vi "main.vi"() -> ()   [LabVIEW 2020]
uses:
  <vilib>/userDefined/High Color/IMAQdx.ctl
  Supporting Files/Sensor Station States.ctl
  Keyence CL-3000/Public/clusters/CL3IF_MEASUREMENT_DATA.ctl
  Keyence CL-3000/Public/clusters/CL3IF_OUTMEASUREMENT_DATA.ctl
  Keyence CL-3000/Public/enums/CL3IF_VALUE_INFO.ctl
  Keyence CL-3000/Public/enums/CL3IF_JUDGE_RESULT.ctl
  Keyence CL-3000/Public/clusters/CL3IF_ETHERNET_SETTING.ctl
  4961857f-4cb1-4452-8877-0132d1278599.vi
  4c07c87f-dbbe-4e69-95de-30caa6fe1779.vi
  8fbe439c-06e5-460e-a560-e938ce784f44.vi
  460a15f0-0b3a-4794-87ef-3f3f720a4f09.vi
  13309ec4-5ddb-4caa-9ccb-149c6c5ba2b7.vi
  762e2a81-f67b-4e5d-a3cd-0f967e3c6027.vi
  <vilib>/Utility/inputDevices.llb/keyboardAcquire.vi
  <vilib>/Utility/inputDevices.llb/closeKeyboard.vi
  Keyence CL-3000/Keyence CL-3000.lvlib
  <vilib>/vision/driver/NI_Vision_Acquisition_Software.lvlib
panel:
  in  "STOP":bool
  in  "Display Tab":enum32{"SENSOR FEEDBACK"}(tab)
  out "Chromatic Confocal":dbl(graph)
  out "Laser Displacement (cRIO)":dbl(graph)
  out "Captured Image":T1(plugin-control)
  out "Camera Feed":T1(plugin-control)
  in  "Motion Tab":enum32{"POSITION", "MEASUREMENT"}(tab)
  in  "Run Program":bool
  in  "Select Program":string(combo)="NONE"
  out "1st Key":T2(ring)
  in  "Bottom Button":bool
  in  "Top Button":bool
  in  "Next Button":bool
  in  "Previous Button":bool
  in  "Up Button":bool
  in  "Down Button":bool
  in  "Jog Axes":bool
  in  "Menu Ring":string(combo)
  in  "Move":bool
  in  "Axis 2 Distance":dbl format="%.2g"
  in  "Axis 1 Distance":dbl format="%.2g"
  in  "Axis 0 Distance":dbl format="%.2g"
  in  "Axis 0 Speed":dbl format="%.2g"
  in  "Axis 1 Speed":dbl format="%.2g"
  in  "Axis 2 Speed":dbl format="%.2g"
  in  "Axis 1 Acc":dbl format="%.2g"
  in  "Axis 0 Acc":dbl format="%.2g"
  in  "Axis 2 Acc":dbl format="%.2g"
  in  "Set Parameters 2":bool
  in  "Axis 2 Jogspeed":dbl format="%.2g"
  in  "Axis 1 Jogspeed":dbl format="%.2g"
  in  "Axis 0 Jogspeed":dbl format="%.2g"
  out "Laser Data Logged":i32
  in  "Capture Image":bool
  in  "Sensor":i32(ring) items=["Chromatic", "Laser"]
  in  "Chromatic Data \nLogging":bool
  out "Chromatic Data Logged":u32
  out "Index End":u32
  out "Index Start":u32
  out "Suffix":string
  in  "Measurement\nAxis":i32(ring) items=["X Axis", "Y Axis"]
  in  "Travel Speed\n(mm/s)":dbl format="%.2g"
  in  "Set Parameters":bool
  in  "Track Offset\n(mm)":dbl format="%.2g"
  in  "Ramp Distance\n(mm)":dbl min=0.0 format="%.2g"
  in  "Num Tracks":i32
  in  "Evaluation Length\n(mm)":dbl max=40.0 format="%.2g"
  in  "Test Name":string
  out "Laser Data\nLogging":bool
  out "Travel Dist":dbl
  in  "Travel Acc\n(mm/s2)":dbl format="%.2g"
  in  "Start Measurement":bool
  in  "Setup Tab":enum32{"SETUP", "MONITORING", "ERRORS"}(tab)
  in  "Home Axes":bool
  in  "Enable Camera":bool
  in  "Enable Laser":bool
  in  "Camera Input":T3
  in  "Enable Chromatic":bool
  in  "IP Address":u8[](array[numeric])=[192, 168, 1, 1]
  in  "Port":u32
  in  "Timeout":u32=5000
  in  "Comm Interface":enum8{"USB", "ETHERNET"}(ring)
  in  "Device ID":i32 min=0 max=2
  out "IsOpen":bool
  in  "Connection?":refnum<k7>(container)
  in  "Connect  to Controller":bool=TRUE
  in  "Set Parameters":bool
  in  "Controller Connection Type":string(combo)="2"
  out "Controller Type":string
  out "Product Name":string
  out "Version":string
  out "Serial Port":fxp<+,3,3>
  in  "Axis Enable":bool
  in  "Save Directory":path
  out "Z Error":bool
  out "Y Error":bool
  out "X Error":bool
  out "Axis 2 Velocity":dbl format="%.3g"
  out "Axis 2 End Pos":dbl format="%.3g"
  out "Axis 2 Position":dbl format="%.3g"
  out "Axis 0 Position":dbl format="%.3f"
  out "Axis 0 End Pos":dbl format="%.3g"
  out "Axis 0 Velocity":dbl format="%.3g"
  out "Axis 1 Position":dbl format="%.3g"
  out "Axis 1 Velocity":dbl format="%.3g"
  out "Axis 1 End Pos":dbl format="%.3g"
  out "A0 Remaining":dbl format="%.3g"
  out "A1 Remaining":dbl format="%.3g"
  out "A2 Remaining":dbl format="%.3g"
  out "Loop Time (us)":u32
  out "Measurement Data":T4(array[cluster])=[{"Out No"=1, "Value"=0, "valueInfo"=enum."VALID", "judgeResult"=0}, {"Out No"=2, "Value"=0, "valueInfo"=enum."VALID", "judgeResult"=0}, {"Out No"=3, "Value"=0, "valueInfo"=enum."VALID", "judgeResult"=0}, {"Out No"=4, "Value"=0, "valueInfo"=enum."VALID", "judgeResult"=0}, {"Out No"=5, "Value"=0, "valueInfo"=enum."VALID", "judgeResult"=0}, {"Out No"=6, "Value"=0, "valueInfo"=enum."VALID", "judgeResult"=0}, {"Out No"=7, "Value"=0, "valueInfo"=enum."VALID", "judgeResult"=0}, {"Out No"=8, "Value"=0, "valueInfo"=enum."VALID", "judgeResult"=0}] {"judgeResult" items=["HI"=1, "GO"=2, "LO"=4, "**"=5, "--"=0]}
  out "Total Time Elapsed (s)":i32
  out "XY Graph":cluster{"X":dbl, "Y":dbl}[](graph)
  out "Controller  Error":errorcluster
  out "Z Axis Error":errorcluster
  out "Y Axis Error":errorcluster
  out "X Axis Error":errorcluster
  out "Chromatic Sensor Error":errorcluster
  # "SET PARAMETERS"
  # "DIRECT MOTION"
  # "SPEED \n(mm/s)"
  # "ACC / DEC\n(mm/s2)"
  # "JOGSPEED \n(mm/s)"
  # "X AXIS"
  # "X AXIS"
  # "(mm)"
  # "Y AXIS"
  # "Y AXIS"
  # "(mm)"
  # "Z AXIS"
  # "Z AXIS"
  # "(mm)"
  # "AXIS JOGGING"
  # "XY AXES"
  # "Z AXIS"
  # "KEYBOARD"
  # "CONTROLLER PROGRAMS"
  # "Suffix will be auto-genereated for each measurement e.g. Test Name_01, Test Name_02, etc."
  # "MEASUREMENT PARAMETERS"
  # "CHROMATIC CONFOCAL"
  # "LASER DISPLACEMENT"
  # "CAMERA"
  # "CONTROLLER SETTINGS"
  # "CHROMATIC CONFOCAL SETTINGS"
  # "LASER DISPLACEMENT SETTINGS"
  # "CAMERA SETTINGS"
  # "AXIS FEEDBACK"
  # "Current Position \n(mm)"
  # "End Position \n(mm)"
  # "Travel Remaining \n(mm)"
  # "Velocity \n(mm/s2)"
  # "X AXIS"
  # "Y AXIS"
  # "Z AXIS"
  # "CONTROLLER"
  # "CHROMATIC CONFOCAL"
  # "CONTROLLER"
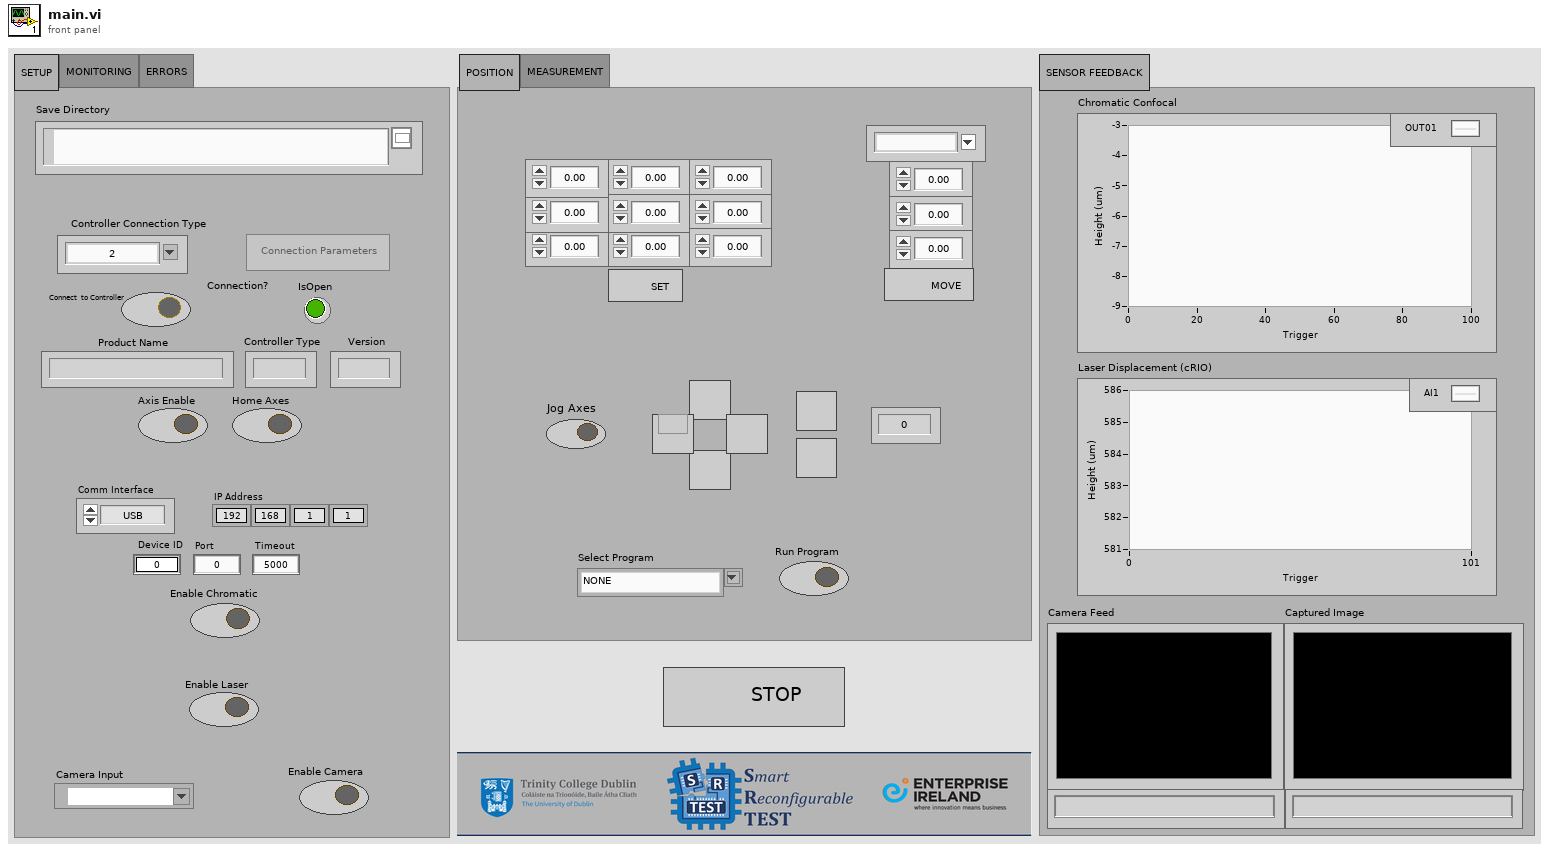
[diagram p1: front panel]
types:
  T1 = typedef "IMAQ Image.ctl" = refnum<image>
  T2 = enum16{"0", "1", "2", "3", "4", "5", "6", "7", "8", "9", "A", "B", "C", "D", "E", "F", "G", "H", "I", "J", "K", "L", "M", "N", "O", "P", "Q", "R", "S", "T", "U", "V", "W", "X", "Y", "Z", "F1", "F2", "F3", "F4", "F5", "F6", "F7", "F8", "F9", "F10", "F11", "F12", "F13", "F14", "F15", "ADD", "BACK", "BACKSLASH", "CAPITAL", "COMMA", "DECIMAL", "DELETE", "DIVIDE", "DOWN", "END", "EQUALS", "ESCAPE", "GRAVE (`)", "HOME", "INSERT", "LBRACKET", "LCONTROL", "LEFT", "L ALT", "LSHIFT", "LWIN", "MINUS", "MULTIPLY", "NEXT", "NUMLOCK", "NUMPAD_0", "NUMPAD_1", "NUMPAD_2", "NUMPAD_3", "NUMPAD_4", "NUMPAD_5", "NUMPAD_6", "NUMPAD_7", "NUMPAD_8", "NUMPAD_9", "PAUSE", "PERIOD", "PRIOR (PG UP)", "RBRACKET", "RCONTROL", "RETURN", "RIGHT", "R ALT", "RSHIFT", "RWIN", "SCROLL", "SEMICOLON", "SLASH", "SPACE", "SUBTRACT", "TAB", "UP", "ENTER (num pad)", "' (quote)"}
  T3 = typedef "IMAQdx.ctl" = refnum<k21>
  T4 = cluster{"Out No":i32, "Value":i32, "valueInfo":enum8{"VALID", "JUDGMENTSTANDBY", "INVALID", "OVERDISPRANGE_P", "OVERDISPRANGE_N"}, "judgeResult":u16}[]
  T5 = enum8{"Enabled", "Disabled", "Disabled and Grayed Out"}
  T6 = enum16{"open", "replace", "create", "open or create", "replace or create", "replace or create with confirmation"}
  T7 = typedef "Sensor Station States.ctl" = enum16{"Initialise", "Acquire", "Visualise", "Log", "Save", "Check Time", "Idle", "Close"}
  T8 = typedef "Keyence CL-3000.lvlib/CL3IF_ETHERNET_SETTING.ctl" = cluster{"IP Address":cluster{"IP1":u8, "IP2":u8, "IP3":u8, "IP4":u8}, "portNo":u32}
  T9 = typedef "Keyence CL-3000.lvlib/CL3IF_MEASUREMENT_DATA.ctl" = cluster{"addInfo":cluster{"triggerCount":u32, "pulseCount":i32}, "outMeasurementData":T10[]}
  T10 = typedef "Keyence CL-3000.lvlib/CL3IF_OUTMEASUREMENT_DATA.ctl" = cluster{"measurementValue":i32, "valueInfo":T11, "judgeResult":T12}
  T11 = typedef "Keyence CL-3000.lvlib/CL3IF_VALUE_INFO.ctl" = enum8{"VALID", "JUDGMENTSTANDBY", "INVALID", "OVERDISPRANGE_P", "OVERDISPRANGE_N"}
  T12 = typedef "Keyence CL-3000.lvlib/CL3IF_JUDGE_RESULT.ctl" = u8
  T13 = enum16{"0", "1", "2", "3", "4", "5", "6", "7", "8", "9", "A", "B", "C", "D", "E", "F", "G", "H", "I", "J", "K", "L", "M", "N", "O", "P", "Q", "R", "S", "T", "U", "V", "W", "X", "Y", "Z", "F1", "F2", "F3", "F4", "F5", "F6", "F7", "F8", "F9", "F10", "F11", "F12", "F13", "F14", "F15", "ADD", "BACK", "BACKSLASH", "CAPITAL", "COMMA", "DECIMAL", "DELETE", "DIVIDE", "DOWN", "END", "EQUALS", "ESCAPE", "GRAVE (`)", "HOME", "INSERT", "LBRACKET", "LCONTROL", "LEFT", "L ALT", "LSHIFT", "LWIN", "MINUS", "MULTIPLY", "NEXT", "NUMLOCK", "NUMPAD_0", "NUMPAD_1", "NUMPAD_2", "NUMPAD_3", "NUMPAD_4", "NUMPAD_5", "NUMPAD_6", "NUMPAD_7", "NUMPAD_8", "NUMPAD_9", "PAUSE", "PERIOD", "PRIOR (PG UP)", "RBRACKET", "RCONTROL", "RETURN", "RIGHT", "R ALT", "RSHIFT", "RWIN", "SCROLL", "SEMICOLON", "SLASH", "SPACE", "SUBTRACT", "TAB", "UP", "ENTER (num pad)", "' (quote)"}[]
  T14 = cluster{"IP Address":u8, "IP Address":u8, "IP Address":u8, "IP Address":u8}
  T15 = cluster{i32, "measurementValue":i32, "valueInfo":T11, "judgeResult":T12}
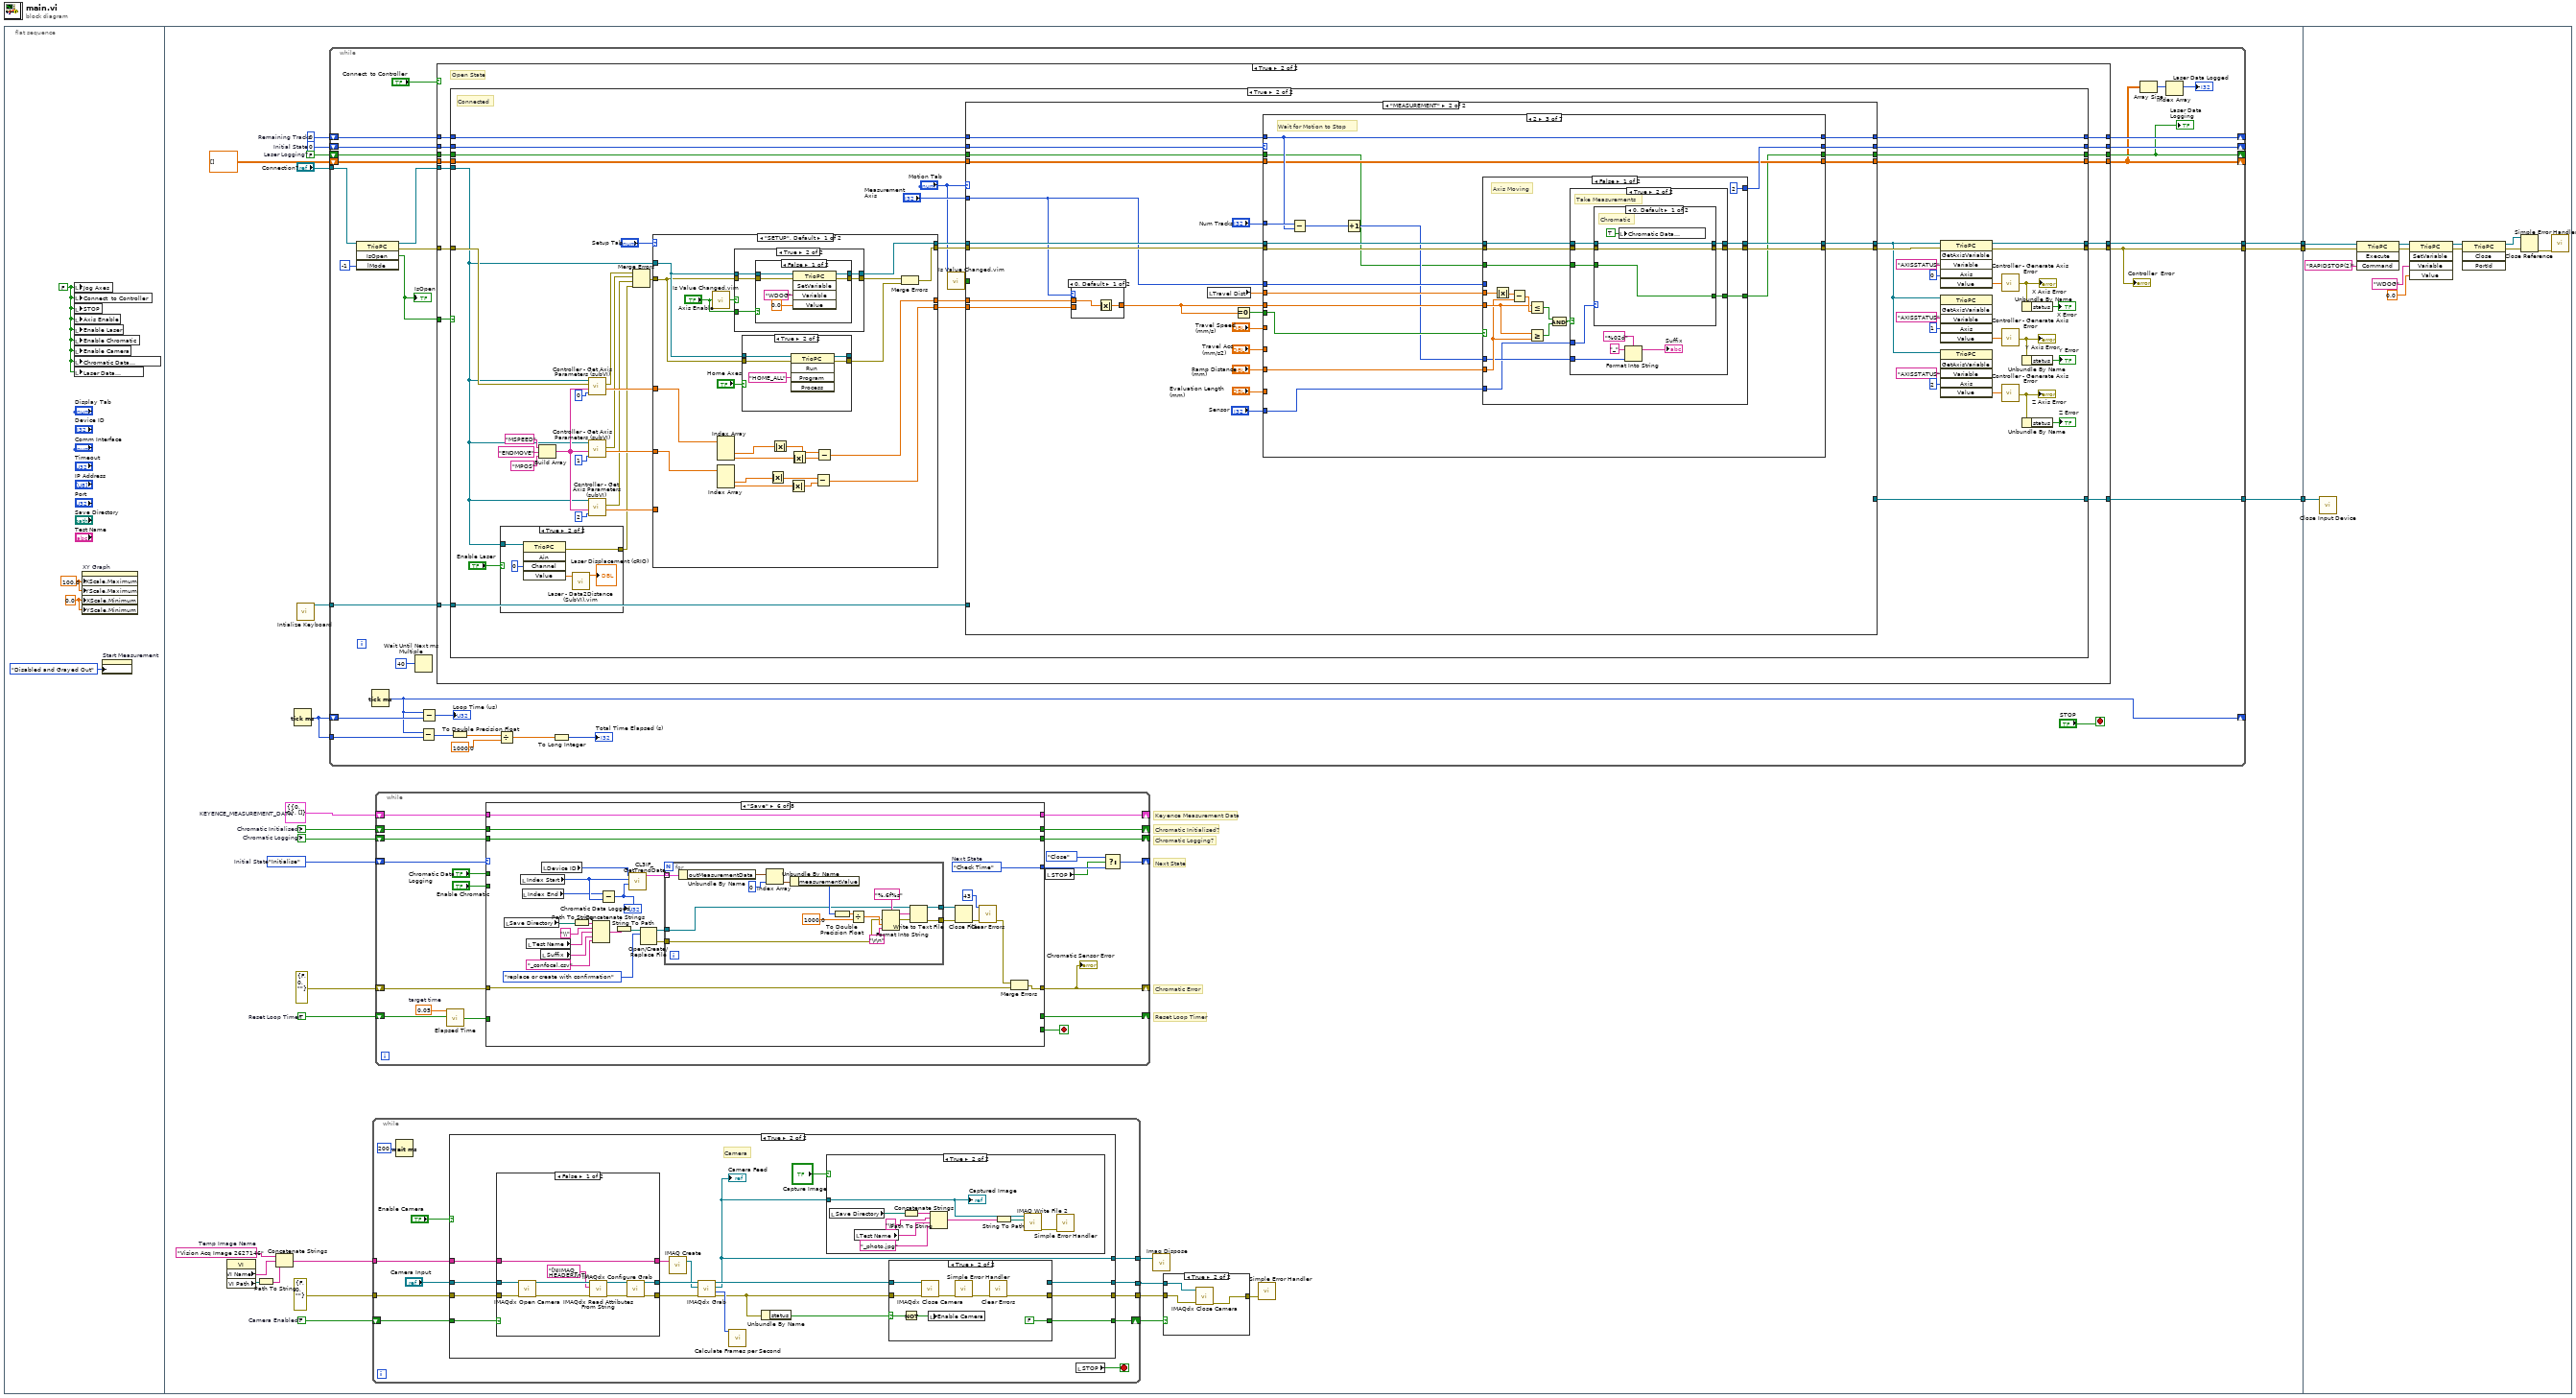
[diagram p0: block diagram]
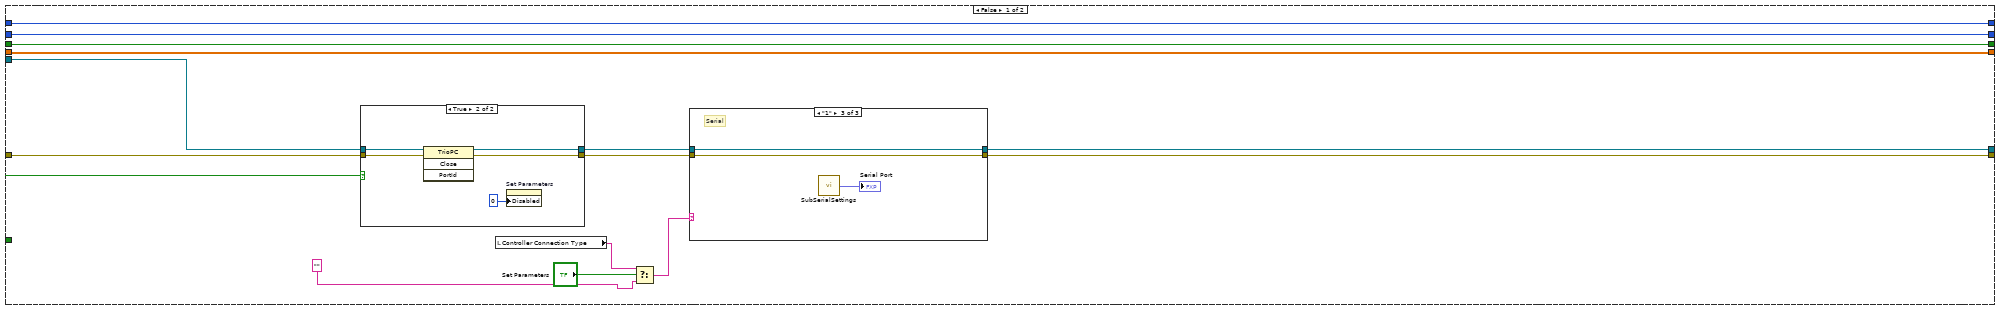
[diagram p2: hidden frame]
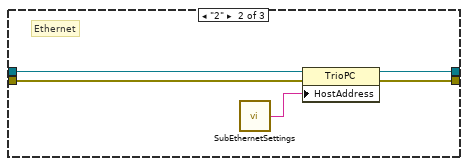
[diagram p5: hidden frame]
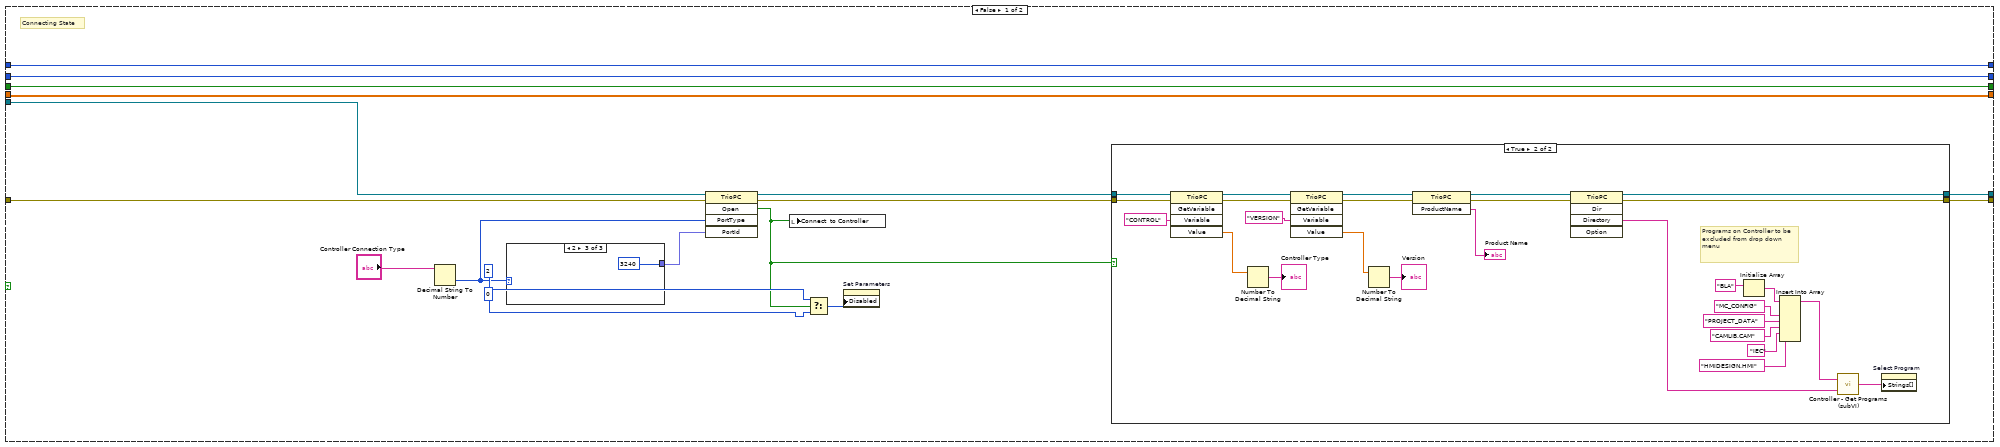
[diagram p6: hidden frame]
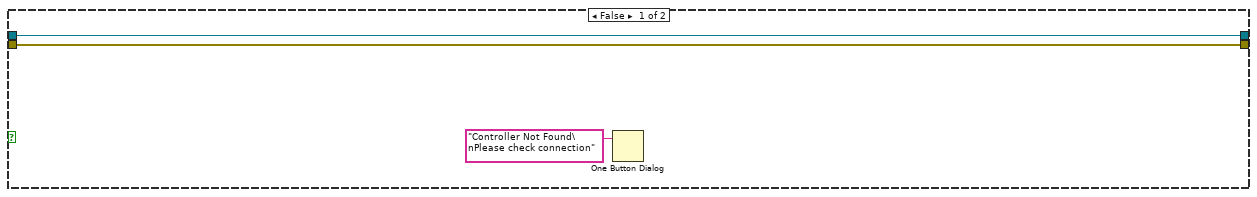
[diagram p7: hidden frame]
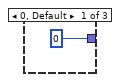
[diagram p8: hidden frame]
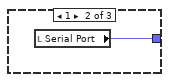
[diagram p9: hidden frame]
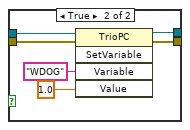
[diagram p13: hidden frame]
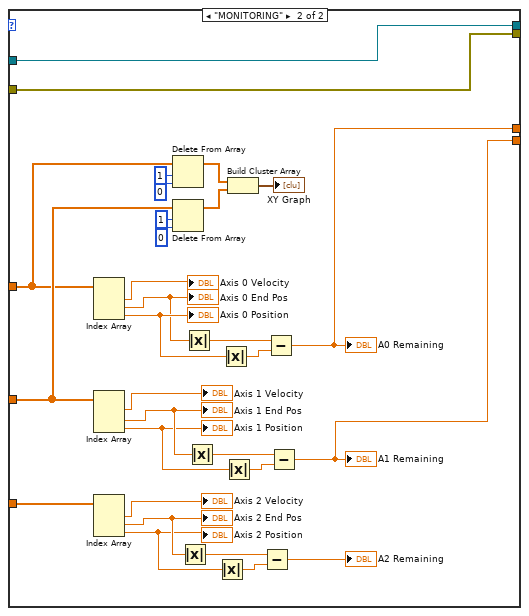
[diagram p14: hidden frame]
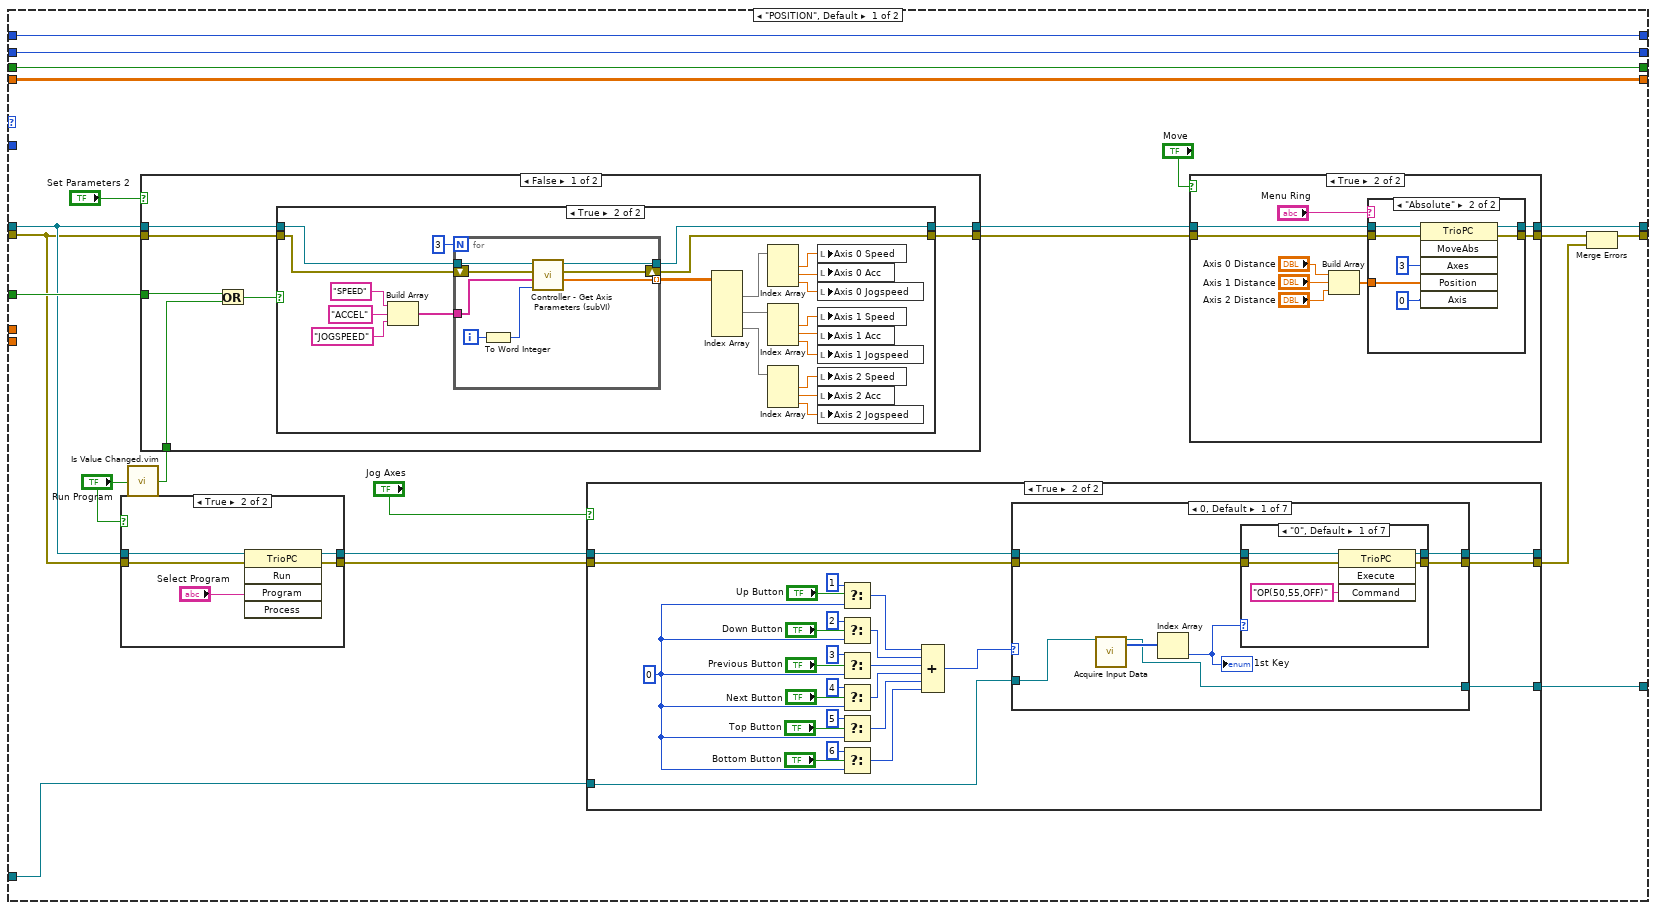
[diagram p15: hidden frame]
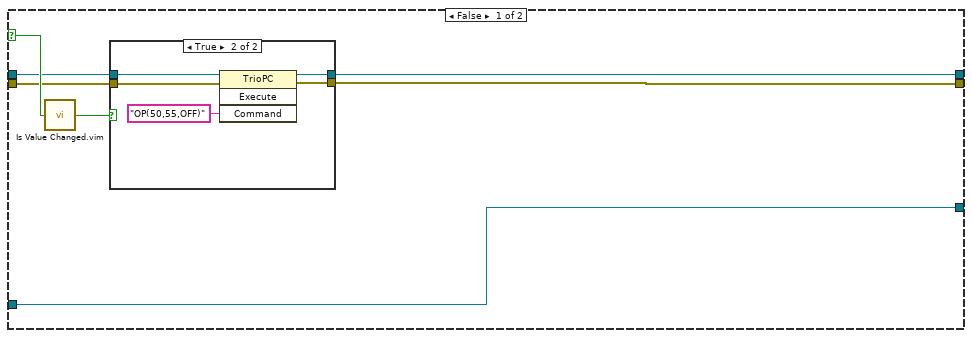
[diagram p17: hidden frame]
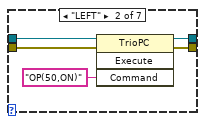
[diagram p19: hidden frame]
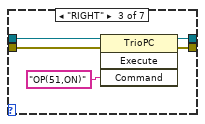
[diagram p20: hidden frame]
diagram:
  n1 = flat-sequence {
    tunnel: [w34] -> w3
    tunnel: [w33] -> w2
    tunnel: [w30] -> w1
    tunnel: w3 -> [w1159]
    tunnel: w2 -> [w1160]
    tunnel: w1 -> [w1161]
    frame #0 {
      w7 = 0.0 ("X Scale.Range:Minimum")
      w6 = 100.0 ("X Scale.Range:Maximum")
      w5 = FALSE ("Jog Axes")
      n2 = local write "Jog Axes"(w5) -> ()
      n3 = local write "Connect  to Controller"(w5) -> ()
      n4 = local write "STOP"(w5) -> ()
      n5 = local write "Axis Enable"(w5) -> ()
      n6 = local write "Enable Laser"(w5) -> ()
      n7 = local write "Enable Chromatic"(w5) -> ()
      n8 = local write "Enable Camera"(w5) -> ()
      n9 = local write "Chromatic Data \nLogging"(w5) -> ()
      n10 = local write "Laser Data\nLogging"(w5) -> ()
      n11 = property on="XY Graph" class="XYGraph (strict)"("XScale.Maximum"=w6, "YScale.Maximum"=w6, "XScale.Minimum"=w7, "YScale.Minimum"=w7) -> ()  [unwired: 2 in, 2 out]
      n12 = property on="Start Measurement" class="Bool"("DisabledEnum"=T5."Disabled and Grayed Out" ("Disabled")) -> ()  [unwired: 2 in, 2 out]
    }
    frame #1 {
      w9 = FALSE  # Laser Logging?
      w10 = 0  # Remaining Tracks
      w11 = 0  # Initial State
      w14 = "Vision Acq Image 2627146"  # Temp Image Name
      w13 = FALSE  # Camera Enabled?
      w24 = FALSE  # Chromatic Initialised?
      w26 = FALSE  # Chromatic Logging?
      w27 = TRUE  # Reset Loop Timer
      w28 = T9 {"addInfo"={"triggerCount"=0, "pulseCount"=0}, "outMeasurementData"=[]}  # KEYENCE_MEASUREMENT_DATA
      w29 = Sensor_Station_States."Initialise"  # Initial State
      # "Reset Loop Timer"
      # "Chromatic Error"
      # "Next State"
      # "Keyence Measurement Data"
      # "Chromatic Logging?"
      # "Chromatic Initialised?"
      n13 = property class="VI"() -> ("VI Name"=w17:string, "VI Path"=w18:path)  [unwired: 2 in, 2 out]
      n14 = Path To String(path=w18) -> (string=w16:string)
      n15 = Concatenate Strings(w14, w17, w16) -> (w19:string)
      n16 = Tick Count (ms)() -> (millisecond timer value=w32:u32)
      n17 = call <vilib>:"Intialize Keyboard.vi"() -> ("device ID"=w31:refnum<k1>)  [unwired: 1 in, 10 out]
      n18 = while {
        tunnel: "Connection?" -> [w65]
        tunnel: [w62] -> w34
        tunnel: [w52] -> w33
        shift-right: [w55] -> _
        shift-left: w32 -> [w58]
        tunnel: w32 -> [w54]
        tunnel: w31 -> [w51]
        tunnel: [w50] -> w30
        shift-right: [w47] -> _
        shift-left: w11 -> [w46]
        shift-right: [w44] -> _
        shift-left: w10 -> [w45]
        shift-right: [w39] -> _
        shift-left: w9 -> [w41]
        shift-right: [w37] -> _
        shift-left: dbl[][] [] ("appended array") -> [w40]
        stop <- "STOP" stop-if-true
        n19 = invoke class="TrioPC" method="IsOpen"(reference=w65, "lMode"=-1) -> (reference out=w49:refnum<k7>, error out=w48:errorcluster, "IsOpen"=w63:bool)  [unwired: 2 in, 1 out]
        "IsOpen" <- w63
        n20 = Tick Count (ms)() -> (millisecond timer value=w55:u32)
        n21 = Wait Until Next ms Multiple(millisecond multiple=u32 40) -> ()  [unwired: 1 out]
        n22 = Subtract(x=w55, y=w54) -> (x-y=w53:u32)
        n23 = Subtract(x=w55, y=w58) -> (x-y=→"Loop Time (us)":u32)
        n24 = case shown="True" "Connect  to Controller" {
          tunnel: [w75 w113] -> w62
          tunnel: [w76 w112] -> w52
          tunnel: w63 -> [w72 w111]
          tunnel: w49 -> [w74 w110]
          tunnel: w48 -> [w73 w109]
          tunnel: w51 -> [_ w108]
          tunnel: [_ w107] -> w50
          tunnel: [w67 w106] -> w47
          tunnel: w46 -> [w67 w105]
          tunnel: w45 -> [w68 w104]
          tunnel: [w68 w103] -> w44
          tunnel: w41 -> [w70 w102]
          tunnel: [w70 w101] -> w39
          tunnel: w40 -> [w69 w100]
          tunnel: [w69 w99] -> w37
          frame False {
            n25 = case shown="True" w72 {
              tunnel: [w83 w88] -> w78
              tunnel: [w82 w87] -> w77
              tunnel: w74 -> [w83 w85]
              tunnel: w73 -> [w82 w84]
              frame False {
              }
              frame True {
                n26 = invoke class="TrioPC" method="Close"(reference=w85, error in=w84) -> (reference out=w88:refnum<k7>, error out=w87:errorcluster)  [unwired: 2 in, 2 out]
                n27 = property on="Set Parameters" class="Bool"("Disabled"=u8 0) -> ()  [unwired: 2 in, 2 out]
              }
            }
            n28 = local read "Controller Connection Type"() -> (w71:string)
            n29 = Select(t=w71, s="Set Parameters", f="") -> (s? t:f=w79:string)
            n30 = case shown="\"1\"" w79 {
              tunnel: w78 -> [w90 w93 w98]
              tunnel: w77 -> [w89 w92 w97]
              tunnel: [w90 w95 w98] -> w75
              tunnel: [w89 w94 w97] -> w76
              frame "", Default {
              }
              frame "2" {
                # "Ethernet"
                n31 = call "SubEthernetSettings.vi"() -> ("Ethernet IP Address 2"=w91:string)
                n32 = property class="TrioPC"(reference=w93, error in=w92, "HostAddress"=w91) -> (reference out=w95:refnum<k7>, error out=w94:errorcluster)
              }
              frame "1" {
                # "Serial"
                n33 = call "SubSerialSettings.vi"() -> ("CommPort"=→"Serial Port":fxp<+,3,3>)
              }
            }
          }
          frame True {
            # "Open State"
            n34 = case shown="True" w111 {
              tunnel: [w121 w208] -> w113
              tunnel: [w122 w201] -> w112
              tunnel: w110 -> [w126 w170]
              tunnel: w109 -> [w125 w179]
              tunnel: w108 -> [_ w218]
              tunnel: [_ w217] -> w107
              tunnel: [w114 w215] -> w106
              tunnel: w105 -> [w114 w214]
              tunnel: w104 -> [w115 w213]
              tunnel: [w115 w212] -> w103
              tunnel: w102 -> [w116 w167]
              tunnel: [w116 w166] -> w101
              tunnel: w100 -> [w117 w165]
              tunnel: [w117 w164] -> w99
              frame False {
                # "Connecting State"
                n35 = Decimal String To Number(string="Controller Connection Type") -> (number=w123:i32)  [unwired: 2 in, 1 out]
                n36 = case shown="2" w123 {
                  tunnel: [i16 0 ("PortId") w162 i16 3240 ("PortId")] -> w130
                  frame 0, Default {
                  }
                  frame 1 {
                    n37 = local read "Serial Port"() -> (w162:fxp<+,3,3>)
                  }
                  frame 2 {
                  }
                }
                n38 = invoke class="TrioPC" method="Open"(reference=w126, error in=w125, "PortType"=w123, "PortId"=w130) -> (reference out=w120:refnum<k7>, error out=w119:errorcluster, "Open"=w118:bool)  [unwired: 1 in, 2 out]
                n39 = local write "Connect  to Controller"(w118) -> ()
                n40 = Select(t=u8 2, s=w118, f=u8 0 ("Disabled")) -> (s? t:f=w127:u8)
                n41 = property on="Set Parameters" class="Bool"("Disabled"=w127) -> ()  [unwired: 2 in, 2 out]
                n42 = case shown="True" w118 {
                  tunnel: [w132 w158] -> w122
                  tunnel: [w133 w157] -> w121
                  tunnel: w120 -> [w133 w148]
                  tunnel: w119 -> [w132 w139]
                  frame False {
                    n43 = One Button Dialog(message="Controller Not Found\nPlease check connection") -> ()  [unwired: 1 in, 1 out]
                  }
                  frame True {
                    # "Programs on Controller to be excluded from drop down menu"
                    n44 = invoke class="TrioPC" method="GetVariable"(reference=w148, error in=w139, "Variable"="CONTROL") -> (reference out=w141:refnum<k7>, error out=w140:errorcluster, "Value"=w145:dbl)  [unwired: 2 in, 2 out]
                    n45 = Number To Decimal String(number=w145) -> (decimal integer string=→"Controller Type":string)  [unwired: 1 in]
                    n46 = invoke class="TrioPC" method="GetVariable"(reference=w141, error in=w140, "Variable"="VERSION") -> (reference out=w137:refnum<k7>, error out=w138:errorcluster, "Value"=w144:dbl)  [unwired: 2 in, 2 out]
                    n47 = Number To Decimal String(number=w144) -> (decimal integer string=→"Version":string)  [unwired: 1 in]
                    n48 = invoke class="TrioPC" method="ProductName"(reference=w137, error in=w138) -> (reference out=w136:refnum<k7>, error out=w135:errorcluster, "ProductName"=→"Product Name":string)  [unwired: 1 in]
                    n49 = invoke class="TrioPC" method="Dir"(reference=w136, error in=w135) -> (reference out=w157:refnum<k7>, error out=w158:errorcluster, "Directory"=w159:string)  [unwired: 3 in, 2 out]
                    n50 = Initialize Array("BLA" ("element")) -> (w156:string[])  [unwired: 1 in]
                    n51 = Insert Into Array(array=w156, new element #1="MC_CONFIG" ("element"), new element #2="PROJECT_DATA" ("element"), new element #3="CAMLIB.CAM" ("element"), new element #4="IEC" ("element"), new element #5="HMIDESIGN.HMI") -> (w149:string[])  [unwired: 1 in]
                    n52 = call "Controller - Get Programs (subVI).vi"("Controller Directory"=w159, "Exclusion List"=w149) -> ("Programs List"=w160:string[])
                    n53 = property on="Select Program" class="CmbBox"("Strings[]"=w160) -> ()  [unwired: 2 in, 2 out]
                  }
                }
              }
              frame True {
                # "Connected"
                n54 = case shown="True" "Enable Laser" {
                  tunnel: w170 -> [_ w223]
                  tunnel: [_ w222] -> w169
                  frame False {
                  }
                  frame True {
                    n55 = invoke class="TrioPC" method="Ain"(reference=w223, "Channel"=i16 0) -> (error out=w222:errorcluster, "Value"=w220:dbl)  [unwired: 3 in, 3 out]
                    n56 = call "Laser - Data2Distance (SubVI).vim"("Raw Data"=w220) -> ("Distance Values"=→"Laser Displacement (cRIO)":dbl)  [unwired: 10 in]
                  }
                }
                n57 = Build Array("MSPEED", "ENDMOVE", "MPOS") -> (w180:string[])
                n58 = call "Controller - Get Axis Parameters (subVI).vi"("Axis"=i16 0, "Axis Parameters"=w180, "error in (no error)"=w179, "Automation Refnum in"=w170) -> ("Axis Parameter Values"=w181:dbl[], "error out"=w178:errorcluster)  [unwired: 5 in, 1 out]
                n59 = call "Controller - Get Axis Parameters (subVI).vi"("Axis"=i16 1, "Axis Parameters"=w180, "Automation Refnum in"=w170) -> ("Axis Parameter Values"=w182:dbl[], "error out"=w177:errorcluster)  [unwired: 6 in, 1 out]
                n60 = call "Controller - Get Axis Parameters (subVI).vi"("Axis"=i16 2, "Axis Parameters"=w180, "Automation Refnum in"=w170) -> ("Axis Parameter Values"=w183:dbl[], "error out"=w176:errorcluster)  [unwired: 6 in, 1 out]
                n61 = Merge Errors(w178, w177, w176, w169) -> (w175:errorcluster)
                n62 = case shown="\"SETUP\", Default" "Setup Tab" {
                  tunnel: w170 -> [w241 w271]
                  tunnel: [w240 w271] -> w174
                  tunnel: [w237 w272] -> w199
                  tunnel: [w224 w276] -> w198
                  tunnel: [w225 w277] -> w191
                  tunnel: w183 -> [_ w275]
                  tunnel: w182 -> [w226 w274]
                  tunnel: w181 -> [w227 w273]
                  tunnel: w175 -> [w236 w272]
                  frame "SETUP", Default {
                    n63 = call "Is Value Changed.vim"("value"="Axis Enable") -> ("changed or first call?"=w243:bool)
                    n64 = Index Array(array=w227) -> (element #2=w232:dbl, element #3=w233:dbl)  [unwired: 3 in, 1 out]
                    n65 = Index Array(array=w226) -> (element #2=w235:dbl, element #3=w234:dbl)  [unwired: 3 in, 1 out]
                    n66 = case shown="True" w243 {
                      tunnel: [w253 w258] -> w239
                      tunnel: w236 -> [w253 w255]
                      tunnel: w241 -> [w252 w257]
                      tunnel: "Axis Enable" -> [_ w256]
                      tunnel: [w252 w254] -> w240
                      frame False {
                      }
                      frame True {
                        n67 = case shown="False" w256 {
                          tunnel: [w260 w266] -> w258
                          tunnel: w255 -> [w261 w267]
                          tunnel: w257 -> [w262 w268]
                          tunnel: [w259 w265] -> w254
                          frame False {
                            n68 = invoke class="TrioPC" method="SetVariable"(reference=w262, error in=w261, "Variable"="WDOG", "Value"=0.0) -> (reference out=w259:refnum<k7>, error out=w260:errorcluster)  [unwired: 1 in, 3 out]
                          }
                          frame True {
                            n69 = invoke class="TrioPC" method="SetVariable"(reference=w268, error in=w267, "Variable"="WDOG", "Value"=1.0) -> (reference out=w265:refnum<k7>, error out=w266:errorcluster)  [unwired: 1 in, 3 out]
                          }
                        }
                      }
                    }
                    n70 = case shown="True" "Home Axes" {
                      tunnel: w241 -> [w246 w250]
                      tunnel: w236 -> [w245 w249]
                      tunnel: [w246 w248] -> _
                      tunnel: [w245 w247] -> w238
                      frame False {
                      }
                      frame True {
                        n71 = invoke class="TrioPC" method="Run"(reference=w250, error in=w249, "Program"="HOME_ALL") -> (reference out=w248:refnum<k7>, error out=w247:errorcluster)  [unwired: 2 in, 3 out]
                      }
                    }
                    n72 = Absolute Value(x=w235) -> (abs(x)=w230:dbl)
                    n73 = Absolute Value(x=w232) -> (abs(x)=w228:dbl)
                    n74 = Absolute Value(x=w234) -> (abs(x)=w231:dbl)
                    n75 = Absolute Value(x=w233) -> (abs(x)=w229:dbl)
                    n76 = Subtract(x=w230, y=w231) -> (x-y=w224:dbl)
                    n77 = Subtract(x=w228, y=w229) -> (x-y=w225:dbl)
                    n78 = Merge Errors(w239, w238) -> (w237:errorcluster)
                  }
                  frame "MONITORING" {
                    n79 = Index Array(array=w273) -> (element #1=→"Axis 0 Velocity":dbl, element #2=w295:dbl, element #3=w296:dbl)  [unwired: 3 in]
                    "Axis 0 Position" <- w296
                    "Axis 0 End Pos" <- w295
                    n80 = Index Array(array=w274) -> (element #1=→"Axis 1 Velocity":dbl, element #2=w299:dbl, element #3=w298:dbl)  [unwired: 3 in]
                    "Axis 1 Position" <- w298
                    "Axis 1 End Pos" <- w299
                    n81 = Index Array(array=w275) -> (element #1=→"Axis 2 Velocity":dbl, element #2=w279:dbl, element #3=w278:dbl)  [unwired: 3 in]
                    "Axis 2 Position" <- w278
                    "Axis 2 End Pos" <- w279
                    n82 = Delete From Array(array=w273, length=1, index=0) -> (array with subset deleted=w288:dbl[])  [unwired: 1 out]
                    n83 = Delete From Array(array=w274, length=1, index=0) -> (array with subset deleted=w287:dbl[])  [unwired: 1 out]
                    n84 = Absolute Value(x=w279) -> (abs(x)=w281:dbl)
                    n85 = Absolute Value(x=w295) -> (abs(x)=w290:dbl)
                    n86 = Absolute Value(x=w299) -> (abs(x)=w292:dbl)
                    n87 = Absolute Value(x=w278) -> (abs(x)=w280:dbl)
                    n88 = Absolute Value(x=w296) -> (abs(x)=w291:dbl)
                    n89 = Absolute Value(x=w298) -> (abs(x)=w293:dbl)
                    n90 = Build Cluster Array(w288, w287) -> (→"XY Graph":cluster{dbl, dbl}[])
                    n91 = Subtract(x=w281, y=w280) -> (x-y=→"A2 Remaining":dbl)
                    n92 = Subtract(x=w290, y=w291) -> (x-y=w277:dbl)
                    "A0 Remaining" <- w277
                    n93 = Subtract(x=w292, y=w293) -> (x-y=w276:dbl)
                    "A1 Remaining" <- w276
                  }
                }
                n94 = call "Is Value Changed.vim"("value"="Motion Tab") -> ("changed or first call?"=w171:bool)
                n95 = case shown="\"MEASUREMENT\"" "Motion Tab" {
                  tunnel: w199 -> [w309 w559]
                  tunnel: [w318 w556] -> w209
                  tunnel: w174 -> [w310 w560]
                  tunnel: [w315 w561] -> w173
                  tunnel: w218 -> [w314 _]
                  tunnel: [w319 _] -> w217
                  tunnel: "Measurement\nAxis" -> [_ w551]
                  tunnel: [w301 w565] -> w215
                  tunnel: w214 -> [w301 w544]
                  tunnel: w213 -> [w302 w564]
                  tunnel: [w302 w563] -> w212
                  tunnel: w191 -> [_ w558]
                  tunnel: w198 -> [_ w557]
                  tunnel: w171 -> [w312 _]
                  tunnel: w167 -> [w304 w546]
                  tunnel: [w304 w545] -> w166
                  tunnel: w165 -> [w303 w543]
                  tunnel: [w303 w542] -> w164
                  frame "POSITION", Default {
                    n96 = case shown="True" "Run Program" {
                      tunnel: w309 -> [w324 w329]
                      tunnel: [w324 w328] -> w307
                      tunnel: w310 -> [w323 w327]
                      tunnel: [w323 w326] -> w308
                      frame False {
                      }
                      frame True {
                        n97 = invoke class="TrioPC" method="Run"(reference=w327, error in=w329, "Program"="Select Program") -> (reference out=w326:refnum<k7>, error out=w328:errorcluster)  [unwired: 2 in, 3 out]
                      }
                    }
                    n98 = call "Is Value Changed.vim"("value"="Run Program") -> ("changed or first call?"=w305:bool)
                    n99 = case shown="False" "Set Parameters 2" {
                      tunnel: [w446 w489] -> w321
                      tunnel: w310 -> [w449 w484]
                      tunnel: w309 -> [w448 w483]
                      tunnel: [w447 w482] -> w322
                      tunnel: w312 -> [w445 _]
                      tunnel: w305 -> [w444 _]
                      frame False {
                        n100 = Or(x=w445, y=w444) -> (x .or. y?=w443:bool)
                        n101 = case shown="True" w443 {
                          tunnel: w449 -> [w451 w468]
                          tunnel: w448 -> [w450 w465]
                          tunnel: [w451 w467] -> w447
                          tunnel: [w450 w466] -> w446
                          frame False {
                          }
                          frame True {
                            n102 = Build Array("SPEED", "ACCEL", "JOGSPEED") -> (w469:string[])
                            n103 = for {
                              N: 3 -> [_]
                              tunnel: w469 -> [w481]
                              tunnel: w468 -> [w480]
                              tunnel: [w477] -> w464 mode=indexing
                              tunnel: [w476] -> w467
                              shift-right: [w475] -> w466
                              shift-left: w465 -> [w474]
                              i -> [w479]
                              n104 = To Word Integer(number=w479) -> (16bit integer=w478:i16)
                              n105 = call "Controller - Get Axis Parameters (subVI).vi"("Axis"=w478, "Axis Parameters"=w481, "error in (no error)"=w474, "Automation Refnum in"=w480) -> ("Axis Parameter Values"=w477:dbl[], "error out"=w475:errorcluster, "Automation Refnum out"=w476:refnum<k7>)  [unwired: 5 in]
                            }
                            n106 = Index Array(array=w464) -> (element #1=w463:dbl[], element #2=w462:dbl[], element #3=w461:dbl[])  [unwired: 6 in]
                            n107 = Index Array(array=w463) -> (element #1=w460:dbl, element #2=w459:dbl, element #3=w458:dbl)  [unwired: 3 in]
                            n108 = Index Array(array=w462) -> (element #1=w456:dbl, element #2=w457:dbl, element #3=w455:dbl)  [unwired: 3 in]
                            n109 = Index Array(array=w461) -> (element #1=w453:dbl, element #2=w454:dbl, element #3=w452:dbl)  [unwired: 3 in]
                            n110 = local write "Axis 0 Speed"(w460) -> ()
                            n111 = local write "Axis 0 Acc"(w459) -> ()
                            n112 = local write "Axis 0 Jogspeed"(w458) -> ()
                            n113 = local write "Axis 1 Speed"(w456) -> ()
                            n114 = local write "Axis 1 Acc"(w457) -> ()
                            n115 = local write "Axis 1 Jogspeed"(w455) -> ()
                            n116 = local write "Axis 2 Speed"(w453) -> ()
                            n117 = local write "Axis 2 Acc"(w454) -> ()
                            n118 = local write "Axis 2 Jogspeed"(w452) -> ()
                          }
                        }
                      }
                      frame True {
                        n119 = Build Array("Axis 0 Speed", "Axis 1 Speed", "Axis 2 Speed") -> (w495:dbl[])
                        n120 = Build Array("Axis 0 Acc", "Axis 1 Acc", "Axis 2 Acc") -> (w494:dbl[])
                        n121 = Build Array("Axis 0 Jogspeed", "Axis 1 Jogspeed", "Axis 2 Jogspeed") -> (w485:dbl[])
                        n122 = for {
                          N: 3 -> [_]
                          tunnel: w495 -> [w507] mode=indexing
                          tunnel: w494 -> [w506] mode=indexing
                          tunnel: w485 -> [w508] mode=indexing
                          shift-right: [w499] -> w489
                          shift-left: w483 -> [w503]
                          shift-right: [w500] -> w482
                          shift-left: w484 -> [w504]
                          i -> [w505]
                          n123 = invoke class="TrioPC" method="SetAxisVariable"(reference=w504, error in=w503, "Variable"="SPEED", "Axis"=w505, "Value"=w507) -> (reference out=w515:refnum<k7>, error out=w514:errorcluster)  [unwired: 1 in, 4 out]
                          n124 = invoke class="TrioPC" method="SetAxisVariable"(reference=w515, error in=w514, "Variable"="ACCEL", "Axis"=w505, "Value"=w506) -> (reference out=w513:refnum<k7>, error out=w512:errorcluster)  [unwired: 1 in, 4 out]
                          n125 = invoke class="TrioPC" method="SetAxisVariable"(reference=w513, error in=w512, "Variable"="DECEL", "Axis"=w505, "Value"=w506) -> (reference out=w502:refnum<k7>, error out=w501:errorcluster)  [unwired: 1 in, 4 out]
                          n126 = invoke class="TrioPC" method="SetAxisVariable"(reference=w502, error in=w501, "Variable"="JOGSPEED", "Axis"=w505, "Value"=w508) -> (reference out=w500:refnum<k7>, error out=w499:errorcluster)  [unwired: 1 in, 4 out]
                        }
                      }
                    }
                    n127 = case shown="True" "Jog Axes" {
                      selector: "Jog Axes" -> [w335 _]
                      tunnel: w314 -> [w336 w347]
                      tunnel: [w336 w346] -> w319
                      tunnel: w308 -> [w333 w349]
                      tunnel: w307 -> [w332 w348]
                      tunnel: [w331 w344] -> w311
                      tunnel: [w330 w345] -> _
                      frame False {
                        n128 = call "Is Value Changed.vim"("value"=w335) -> ("changed or first call?"=w334:bool)
                        n129 = case shown="True" w334 {
                          tunnel: [w338 w342] -> w330
                          tunnel: [w337 w341] -> w331
                          tunnel: w333 -> [w338 w340]
                          tunnel: w332 -> [w337 w339]
                          frame False {
                          }
                          frame True {
                            n130 = invoke class="TrioPC" method="Execute"(reference=w340, error in=w339, "Command"="OP(50,55,OFF)") -> (reference out=w342:refnum<k7>, error out=w341:errorcluster)  [unwired: 1 in, 2 out]
                          }
                        }
                      }
                      frame True {
                        w356 = 0 ("f")
                        n131 = Select(t=1, s="Up Button", f=w356) -> (s? t:f=w363:i32)
                        n132 = Select(t=2, s="Down Button", f=w356) -> (s? t:f=w362:i32)
                        n133 = Select(t=3, s="Previous Button", f=w356) -> (s? t:f=w361:i32)
                        n134 = Select(t=4, s="Next Button", f=w356) -> (s? t:f=w360:i32)
                        n135 = Select(t=5, s="Top Button", f=w356) -> (s? t:f=w359:i32)
                        n136 = Select(t=6, s="Bottom Button", f=w356) -> (s? t:f=w358:i32)
                        n137 = Compound Arithmetic op=ADD(w363, w362, w361, w360, w359, w358) -> (w357:i32)
                        n138 = case shown="0, Default" w357 {
                          tunnel: w349 -> [w375 w416 w422 w426 w432 w437 w442]
                          tunnel: w348 -> [w374 w415 w421 w427 w431 w436 w441]
                          tunnel: [w373 w413 w420 w425 w430 w435 w440] -> w345
                          tunnel: [w372 w414 w419 w424 w429 w434 w439] -> w344
                          tunnel: w347 -> [w371 _ _ _ _ _ _]
                          tunnel: [w370 _ _ _ _ _ _] -> w346
                          frame 0, Default {
                            n139 = call-poly <vilib>:"Acquire Input Data.vi"("device ID"=w371) -> ("device ID"=w370:refnum<k1>, "keys pressed"=w376:T13)  [unwired: 1 in, 16 out]
                            n140 = Index Array(array=w376) -> (element=w377:T2)  [unwired: 1 in]
                            "1st Key" <- w377
                            n141 = case shown="\"0\", Default" w377 {
                              tunnel: w375 -> [w382 w386 w392 w396 w402 w407 w412]
                              tunnel: w374 -> [w381 w387 w391 w395 w401 w406 w411]
                              tunnel: [w380 w385 w390 w393 w400 w405 w410] -> w373
                              tunnel: [w379 w384 w389 w394 w399 w404 w409] -> w372
                              frame "0", Default {
                                n142 = invoke class="TrioPC" method="Execute"(reference=w382, error in=w381, "Command"="OP(50,55,OFF)") -> (reference out=w380:refnum<k7>, error out=w379:errorcluster)  [unwired: 1 in, 2 out]
                              }
                              frame "LEFT" {
                                n143 = invoke class="TrioPC" method="Execute"(reference=w386, error in=w387, "Command"="OP(50,ON)") -> (reference out=w385:refnum<k7>, error out=w384:errorcluster)  [unwired: 1 in, 2 out]
                              }
                              frame "RIGHT" {
                                n144 = invoke class="TrioPC" method="Execute"(reference=w392, error in=w391, "Command"="OP(51,ON)") -> (reference out=w390:refnum<k7>, error out=w389:errorcluster)  [unwired: 1 in, 2 out]
                              }
                              frame "UP" {
                                n145 = invoke class="TrioPC" method="Execute"(reference=w396, error in=w395, "Command"="OP(53,ON)") -> (reference out=w393:refnum<k7>, error out=w394:errorcluster)  [unwired: 1 in, 2 out]
                              }
                              frame "DOWN" {
                                n146 = invoke class="TrioPC" method="Execute"(reference=w402, error in=w401, "Command"="OP(52,ON)") -> (reference out=w400:refnum<k7>, error out=w399:errorcluster)  [unwired: 1 in, 2 out]
                              }
                              frame "PRIOR (PG UP)" {
                                n147 = invoke class="TrioPC" method="Execute"(reference=w407, error in=w406, "Command"="OP(54,ON)") -> (reference out=w405:refnum<k7>, error out=w404:errorcluster)  [unwired: 1 in, 2 out]
                              }
                              frame "NEXT" {
                                n148 = invoke class="TrioPC" method="Execute"(reference=w412, error in=w411, "Command"="OP(55,ON)") -> (reference out=w410:refnum<k7>, error out=w409:errorcluster)  [unwired: 1 in, 2 out]
                              }
                            }
                          }
                          frame 1 {
                            n149 = invoke class="TrioPC" method="Execute"(reference=w416, error in=w415, "Command"="OP(53,ON)") -> (reference out=w413:refnum<k7>, error out=w414:errorcluster)  [unwired: 1 in, 2 out]
                          }
                          frame 2 {
                            n150 = invoke class="TrioPC" method="Execute"(reference=w422, error in=w421, "Command"="OP(52,ON)") -> (reference out=w420:refnum<k7>, error out=w419:errorcluster)  [unwired: 1 in, 2 out]
                          }
                          frame 3 {
                            n151 = invoke class="TrioPC" method="Execute"(reference=w426, error in=w427, "Command"="OP(50,ON)") -> (reference out=w425:refnum<k7>, error out=w424:errorcluster)  [unwired: 1 in, 2 out]
                          }
                          frame 4 {
                            n152 = invoke class="TrioPC" method="Execute"(reference=w432, error in=w431, "Command"="OP(51,ON)") -> (reference out=w430:refnum<k7>, error out=w429:errorcluster)  [unwired: 1 in, 2 out]
                          }
                          frame 5 {
                            n153 = invoke class="TrioPC" method="Execute"(reference=w437, error in=w436, "Command"="OP(54,ON)") -> (reference out=w435:refnum<k7>, error out=w434:errorcluster)  [unwired: 1 in, 2 out]
                          }
                          frame 6 {
                            n154 = invoke class="TrioPC" method="Execute"(reference=w442, error in=w441, "Command"="OP(55,ON)") -> (reference out=w440:refnum<k7>, error out=w439:errorcluster)  [unwired: 1 in, 2 out]
                          }
                        }
                      }
                    }
                    n155 = case shown="True" "Move" {
                      tunnel: [w518 w520] -> w315
                      tunnel: [w517 w519] -> w316
                      tunnel: w322 -> [w518 w523]
                      tunnel: w321 -> [w517 w522]
                      frame False {
                      }
                      frame True {
                        n156 = Build Array("Axis 0 Distance", "Axis 1 Distance", "Axis 2 Distance") -> (w521:dbl[])
                        n157 = case shown="\"Absolute\"" "Menu Ring" {
                          tunnel: w523 -> [w534 w540]
                          tunnel: w522 -> [w533 w539]
                          tunnel: w521 -> [w531 w536]
                          tunnel: [w529 w537] -> w520
                          tunnel: [w528 w538] -> w519
                          frame "Relative", Default {
                            n158 = invoke class="TrioPC" method="MoveRel"(reference=w534, error in=w533, "Axes"=i16 3, "Distance"=w531, "Axis"=0) -> (reference out=w529:refnum<k7>, error out=w528:errorcluster)  [unwired: 1 in, 4 out]
                          }
                          frame "Absolute" {
                            n159 = invoke class="TrioPC" method="MoveAbs"(reference=w540, error in=w539, "Axes"=i16 3, "Position"=w536, "Axis"=i16 0 ("Axes")) -> (reference out=w537:refnum<k7>, error out=w538:errorcluster)  [unwired: 1 in, 4 out]
                          }
                        }
                      }
                    }
                    n160 = Merge Errors(w316, w311) -> (w318:errorcluster)
                  }
                  frame "MEASUREMENT" {
                    n161 = case shown="0, Default" w551 {
                      tunnel: w558 -> [w567 _]
                      tunnel: w557 -> [_ w569]
                      tunnel: [w566 w568] -> w549
                      frame 0, Default {
                        n162 = Absolute Value(x=w567) -> (abs(x)=w566:dbl)
                      }
                      frame 1 {
                        n163 = Absolute Value(x=w569) -> (abs(x)=w568:dbl)
                      }
                    }
                    n164 = local read "Travel Dist"() -> (w562:dbl)
                    n165 = Equal To 0?(x=w549) -> (x = 0?=w550:bool)
                    n166 = case shown="2" w544 {
                      tunnel: w560 -> [w577 w641 w684 w797 w804 w842 w864]
                      tunnel: w559 -> [w576 w642 w685 w796 w803 w841 w863]
                      tunnel: w551 -> [_ w640 w686 w787 _ _ _]
                      tunnel: [w579 w639 w682 w794 w801 w833 w868] -> w556
                      tunnel: [w578 w638 w683 w795 w802 w834 w864] -> w561
                      tunnel: [w584 w636 w690 4 ("Measurement\nAxis") w805 3 ("Measurement\nAxis") 0 ("Axes")] -> w565
                      tunnel: w564 -> [_ w635 w680 w785 w807 w829 w865]
                      tunnel: [w583 w635 w680 w785 w806 w829 w865] -> w563
                      tunnel: w550 -> [_ _ w691 _ w808 _ _]
                      tunnel: w549 -> [_ _ w689 _ _ _ _]
                      tunnel: "Ramp Distance\n(mm)" -> [w575 w633 w688 _ _ _ _]
                      tunnel: w562 -> [_ w634 w687 w784 _ _ _]
                      tunnel: "Travel Acc\n(mm/s2)" -> [w582 _ _ _ _ _ _]
                      tunnel: "Travel Speed\n(mm/s)" -> [w581 _ _ _ w800 _ _]
                      tunnel: "Evaluation Length\n(mm)" -> [w580 _ _ _ _ _ _]
                      tunnel: "Num Tracks" -> [w573 _ w681 _ _ _ _]
                      tunnel: "Sensor" -> [_ _ w677 _ _ _ _]
                      tunnel: w546 -> [w571 w631 w675 w782 w798 w831 w893]
                      tunnel: [w571 w630 w674 w782 w798 w831 w893] -> w545
                      tunnel: w543 -> [w570 w629 w676 w783 w799 w843 w874]
                      tunnel: [w570 w629 w676 w783 w799 w832 dbl[][] [] ("appended array")] -> w542
                      frame 0, Default {
                        # "Not Measuring"
                        n167 = case shown="True" "Set Parameters" {
                          tunnel: [w591 w613] -> w578
                          tunnel: [w590 w612] -> w579
                          tunnel: w577 -> [w591 w598]
                          tunnel: w576 -> [w590 w597]
                          tunnel: w582 -> [_ w608]
                          tunnel: w581 -> [_ w607]
                          tunnel: w580 -> [_ w601]
                          tunnel: w575 -> [_ w606]
                          frame False {
                          }
                          frame True {
                            n168 = invoke class="TrioPC" method="Execute"(reference=w598, error in=w597, "Command"="NEW \"TABLE\"") -> (reference out=w596:refnum<k7>, error out=w595:errorcluster)  [unwired: 1 in, 2 out]
                            n169 = Absolute Value(x=w606) -> (abs(x)=w610:dbl)
                            n170 = Absolute Value(x=w601) -> (abs(x)=w605:dbl)
                            n171 = Multiply(x=w610, y=2.0) -> (x*y=w604:dbl)
                            n172 = invoke class="TrioPC" method="Execute"(reference=w596, error in=w595, "Command"="SCOPE(ON,20,0,3000,MPOS AXIS(0),MPOS AXIS(1),AIN(0))") -> (reference out=w593:refnum<k7>, error out=w592:errorcluster)  [unwired: 1 in, 2 out]
                            n173 = Add(x=w604, y=w605) -> (x+y=w603:dbl)
                            n174 = Sign(1:w601) -> (0:w602:dbl)
                            n175 = Multiply(x=w603, y=w602) -> (x*y=→"Travel Dist":dbl)
                            n176 = for {
                              N: 2 -> [_]
                              tunnel: w607 -> [w621]
                              tunnel: w608 -> [w620]
                              shift-right: [w615] -> w612
                              shift-left: w592 -> [w617]
                              shift-right: [w616] -> w613
                              shift-left: w593 -> [w618]
                              i -> [w619]
                              n177 = invoke class="TrioPC" method="SetAxisVariable"(reference=w618, error in=w617, "Variable"="SPEED", "Axis"=w619, "Value"=w621) -> (reference out=w627:refnum<k7>, error out=w626:errorcluster)  [unwired: 1 in, 4 out]
                              n178 = invoke class="TrioPC" method="SetAxisVariable"(reference=w627, error in=w626, "Variable"="ACCEL", "Axis"=w619, "Value"=w620) -> (reference out=w625:refnum<k7>, error out=w624:errorcluster)  [unwired: 1 in, 4 out]
                              n179 = invoke class="TrioPC" method="SetAxisVariable"(reference=w625, error in=w624, "Variable"="DECEL", "Axis"=w619, "Value"=w620) -> (reference out=w616:refnum<k7>, error out=w615:errorcluster)  [unwired: 1 in, 4 out]
                            }
                            n180 = property on="Start Measurement" class="Bool"("DisabledEnum"=T5."Enabled" ("Disabled")) -> ()  [unwired: 2 in, 2 out]
                          }
                        }
                        n181 = case shown="True" "Start Measurement" {
                          tunnel: [0 ("Axes") 1 ("Axes")] -> w584
                          tunnel: [0 ("f") w589] -> w583
                          tunnel: w573 -> [_ w589]
                          frame False {
                          }
                          frame True {
                            n182 = local write "Setup Tab"(enum32{"SETUP", "MONITORING", "ERRORS"}."MONITORING" ("Setup Tab")) -> ()
                          }
                        }
                      }
                      frame 1 {
                        # "Start Measurement Sequence"
                        n183 = Equal To 0?(x=w633) -> (x = 0?=w632:bool)
                        n184 = Not Equal To 0?(x=w635) -> (x != 0?=w637:bool)
                        n185 = case shown="False" w637 {
                          tunnel: w642 -> [w652 w665]
                          tunnel: w641 -> [w653 w664]
                          tunnel: w640 -> [_ w663]
                          tunnel: [w652 w656] -> w639
                          tunnel: [w653 w657] -> w638
                          tunnel: [w643 2 ("Axes")] -> w636
                          tunnel: w634 -> [_ w660]
                          tunnel: w632 -> [_ w655]
                          tunnel: w631 -> [w651 _]
                          tunnel: [w651 w654] -> w630
                          tunnel: w629 -> [w647 _]
                          frame False {
                            # "Save Laser Data"
                            # "Return to Idle State"
                            # "No Tracks to measure"
                            n186 = Array Size(array=w647) -> (size(s)=w650:i32[])
                            n187 = Index Array(array=w650, index=0) -> (element=w649:i32)
                            n188 = Equal To 0?(x=w649) -> (x = 0?=w645:bool)
                            n189 = Select(t=0 ("Axes"), s=w645, f=6) -> (s? t:f=w643:i32)
                          }
                          frame True {
                            n190 = invoke class="TrioPC" method="MoveRel"(reference=w664, error in=w665, "Axes"=i16 1, "Distance"=w660, "Axis"=w663) -> (reference out=w659:refnum<k7>, error out=w658:errorcluster)  [unwired: 1 in, 4 out]
                            n191 = case shown="True" w655 {
                              tunnel: w659 -> [w667 w673]
                              tunnel: w658 -> [w666 w672]
                              tunnel: [w667 w671] -> w657
                              tunnel: [w666 w670] -> w656
                              tunnel: [FALSE TRUE] -> w654
                              frame False {
                              }
                              frame True {
                                # "No Ramp Distance"
                                n192 = invoke class="TrioPC" method="Trigger"(reference=w673, error in=w672) -> (reference out=w671:refnum<k7>, error out=w670:errorcluster)  [unwired: 1 in, 1 out]
                              }
                            }
                          }
                        }
                      }
                      frame 2 {
                        # "Wait for Motion to Stop"
                        n193 = Subtract(x=w681, y=w680) -> (x-y=w679:i32)
                        n194 = Increment(x=w679) -> (x+1=w678:i32)
                        n195 = case shown="False" w691 {
                          tunnel: [2 ("Measurement\nAxis") w764] -> w690
                          tunnel: w689 -> [w706 _]
                          tunnel: w688 -> [w705 _]
                          tunnel: w687 -> [w701 _]
                          tunnel: w686 -> [_ _]
                          tunnel: w685 -> [w693 w770]
                          tunnel: w684 -> [w694 w772]
                          tunnel: [w695 w769] -> w683
                          tunnel: [w696 w768] -> w682
                          tunnel: w678 -> [w699 _]
                          tunnel: w677 -> [w698 w765]
                          tunnel: w675 -> [w697 _]
                          tunnel: [w692 FALSE ("Laser Data\nLogging")] -> w674
                          frame False {
                            # "Axis Moving"
                            n196 = Absolute Value(x=w701) -> (abs(x)=w700:dbl)
                            n197 = Subtract(x=w700, y=w705) -> (x-y=w707:dbl)
                            n198 = Less Or Equal?(x=w706, y=w707) -> (x <= y?=w704:bool)
                            n199 = Greater Or Equal?(x=w706, y=w705) -> (x >= y?=w703:bool)
                            n200 = And(x=w704, y=w703) -> (x .and. y?=w702:bool)
                            n201 = case shown="True" w702 {
                              tunnel: w699 -> [_ w745]
                              tunnel: w698 -> [w715 w741]
                              tunnel: w697 -> [w714 w736]
                              tunnel: [w713 w737] -> w696
                              tunnel: [w712 w739] -> w695
                              tunnel: w694 -> [w711 w740]
                              tunnel: w693 -> [w710 w738]
                              tunnel: [w709 w735] -> w692
                              frame False {
                                # "Axis Ramping Up / Down"
                                n202 = case shown="0, Default" w715 {
                                tunnel: w714 -> [w716 w723]
                                tunnel: [w717 w725] -> w713
                                tunnel: [w718 w724] -> w712
                                tunnel: w711 -> [w718 w722]
                                tunnel: w710 -> [w717 w721]
                                tunnel: [w716 w720] -> w709
                                frame 0, Default {
                                # "Chromatic"
                                n203 = local write "Chromatic Data \nLogging"(FALSE ("Log Chromatic Data")) -> ()
                                }
                                frame 1 {
                                # "Laser"
                                n204 = case shown="True" w723 {
                                selector: w723 -> [w728 _]
                                tunnel: [w726 w733] -> w725
                                tunnel: [w727 w732] -> w724
                                tunnel: w722 -> [w727 w731]
                                tunnel: w721 -> [w726 w730]
                                tunnel: [w728 FALSE ("Log Chromatic Data")] -> w720
                                frame False {
                                # "Axis Ramping Up"
                                }
                                frame True {
                                # "Axis Ramping Down"
                                n205 = invoke class="TrioPC" method="Execute"(reference=w731, error in=w730, "Command"="SCOPE(OFF)") -> (reference out=w732:refnum<k7>, error out=w733:errorcluster)  [unwired: 1 in, 2 out]
                                }
                                }
                                }
                                }
                              }
                              frame True {
                                # "Take Measurements"
                                n206 = case shown="0, Default" w741 {
                                tunnel: [w748 w753] -> w739
                                tunnel: w740 -> [w748 w755]
                                tunnel: w738 -> [w747 w754]
                                tunnel: [w747 w752] -> w737
                                tunnel: w736 -> [w746 w751]
                                tunnel: [w746 w750] -> w735
                                frame 0, Default {
                                # "Chromatic"
                                n207 = local write "Chromatic Data \nLogging"(TRUE ("Log Chromatic Data")) -> ()
                                }
                                frame 1 {
                                # "Laser"
                                n208 = case shown="False" w751 {
                                selector: w751 -> [_ w763]
                                tunnel: w755 -> [w760 w761]
                                tunnel: w754 -> [w759 w762]
                                tunnel: [w758 w761] -> w753
                                tunnel: [w757 w762] -> w752
                                tunnel: [TRUE ("Log Chromatic Data") w763] -> w750
                                frame False {
                                # "Start measurement"
                                n209 = invoke class="TrioPC" method="Trigger"(reference=w760, error in=w759) -> (reference out=w758:refnum<k7>, error out=w757:errorcluster)  [unwired: 1 in, 1 out]
                                }
                                frame True {
                                # "Measuring..."
                                }
                                }
                                }
                                }
                                n210 = Format Into String(format string="%02d", initial string="_", w745) -> (resulting string=→"Suffix":string)  [unwired: 1 in, 1 out]
                              }
                            }
                          }
                          frame True {
                            # "For instances when no ramp distance specified"
                            # "Increase speed for return motion"
                            # "Track Movement Finished"
                            n211 = for {
                              N: 2 -> [_]
                              tunnel: w772 -> [w780]
                              tunnel: [w776] -> w769
                              shift-right: [w775] -> w768
                              shift-left: w770 -> [w781]
                              i -> [w779]
                              n212 = invoke class="TrioPC" method="SetAxisVariable"(reference=w780, error in=w781, "Variable"="SPEED", "Axis"=w779, "Value"=5.0) -> (reference out=w776:refnum<k7>, error out=w775:errorcluster)  [unwired: 1 in, 4 out]
                            }
                            n213 = local write "Chromatic Data \nLogging"(FALSE ("Chromatic Data \nLogging")) -> ()
                            n214 = case shown="0, Default" w765 {
                              tunnel: [3 ("Measurement\nAxis") 5 ("Measurement\nAxis")] -> w764
                              frame 0, Default {
                                # "Chromatic"
                              }
                              frame 1 {
                                # "Laser"
                              }
                            }
                          }
                        }
                      }
                      frame 3 {
                        # "Return to start position / start of next track"
                        n215 = Build Array("Track Offset\n(mm)") -> (w791:dbl[])
                        n216 = Negate(x=w784) -> (-x=w792:dbl)
                        n217 = Insert Into Array(array=w791, index=w787, new element=w792) -> (w790:dbl[])
                        n218 = invoke class="TrioPC" method="MoveRel"(reference=w797, error in=w796, "Axes"=i16 2, "Distance"=w790, "Axis"=i16 0 ("Axes")) -> (reference out=w795:refnum<k7>, error out=w794:errorcluster)  [unwired: 1 in, 4 out]
                      }
                      frame 4 {
                        # "Wait until returned and axes stopped"
                        n219 = case shown="True" w808 {
                          tunnel: w807 -> [w812 w821]
                          tunnel: [w812 w820] -> w806
                          tunnel: [4 ("Measurement\nAxis") 1 ("Measurement\nAxis")] -> w805
                          tunnel: w804 -> [w810 w817]
                          tunnel: w803 -> [w809 w816]
                          tunnel: [w810 w815] -> w802
                          tunnel: [w809 w814] -> w801
                          tunnel: w800 -> [_ w813]
                          frame False {
                            # "Still Moving"
                          }
                          frame True {
                            # "Start next measurement"
                            # "Finished Movement"
                            n220 = for {
                              N: 2 -> [_]
                              tunnel: w817 -> [w827]
                              tunnel: [w824] -> w815
                              shift-right: [w823] -> w814
                              shift-left: w816 -> [w828]
                              tunnel: w813 -> [w822]
                              i -> [w826]
                              n221 = invoke class="TrioPC" method="SetAxisVariable"(reference=w827, error in=w828, "Variable"="SPEED", "Axis"=w826, "Value"=w822) -> (reference out=w824:refnum<k7>, error out=w823:errorcluster)  [unwired: 1 in, 4 out]
                            }
                            n222 = Decrement(x=w821) -> (x-1=w820:i32)
                          }
                        }
                      }
                      frame 5 {
                        w857 = 1000 ("index")
                        w860 = 3000 ("PortId")
                        # "If using laser - Retreive stored data from controller and reset logging"
                        n223 = Initialize Array(0.0 ("disabled index (col)"), w860) -> (w850:dbl[])
                        n224 = invoke class="TrioPC" method="GetTable"(reference=w842, error in=w841, "StartPosition"=0 ("PortId"), "NumberOfValues"=w860, "Values"=w850) -> (reference out=w840:refnum<k7>, error out=w839:errorcluster, "Values"=w851:variant)  [unwired: 1 in, 3 out]
                        n225 = Variant To Data(type=w850, Variant=w851) -> (data=w859:dbl[])  [unwired: 1 in, 1 out]
                        n226 = Split 1D Array(array=w859, index=w857) -> (first subarray=w856:dbl[], second subarray=w858:dbl[])
                        n227 = Split 1D Array(array=w858, index=w857) -> (first subarray=w854:dbl[], second subarray=w852:dbl[])
                        n228 = Search 1D Array(1D array=w852, element=0.0) -> (index of element=w855:i32)  [unwired: 1 in]
                        n229 = Split 1D Array(array=w856, index=w855) -> (first subarray=w849:dbl[])  [unwired: 1 out]
                        n230 = Split 1D Array(array=w854, index=w855) -> (first subarray=w848:dbl[])  [unwired: 1 out]
                        n231 = Split 1D Array(array=w852, index=w855) -> (first subarray=w847:dbl[])  [unwired: 1 out]
                        n232 = call "Laser - Data2Distance (SubVI).vim"("Raw Data"=w847) -> ("Distance Values"=w846:dbl[])  [unwired: 10 in]
                        n233 = Build Array(w849, w848, w846) -> (w845:dbl[][])
                        n234 = Transpose 2D Array(2D array=w845) -> (transposed array=w844:dbl[][])
                        n235 = invoke class="TrioPC" method="Execute"(reference=w840, error in=w839, "Command"="NEW \"TABLE\"") -> (reference out=w836:refnum<k7>, error out=w835:errorcluster)  [unwired: 1 in, 2 out]
                        n236 = Build Array (concatenate)(w843, w844) -> (w832:dbl[][])
                        n237 = invoke class="TrioPC" method="Execute"(reference=w836, error in=w835, "Command"="SCOPE(ON,20,0,3000,MPOS AXIS(0),MPOS AXIS(1),AIN(0))") -> (reference out=w834:refnum<k7>, error out=w833:errorcluster)  [unwired: 1 in, 2 out]
                      }
                      frame 6 {
                        # "If using laser - Save recorded data"
                        n238 = local read "Save Directory"() -> (w889:path)
                        n239 = local read "Test Name"() -> (w885:string)
                        n240 = Path To String(path=w889) -> (string=w888:string)
                        n241 = Concatenate Strings(w888, "\\" ("string"), w885, "_laser.csv" ("string")) -> (w887:string)
                        n242 = String To Path(string=w887) -> (path=w886:path)
                        n243 = Array To Spreadsheet String(delimiter (Tab)=",", array=string[] ["X Position (cm)", "Y Position (cm)", "Height (um)"], 3:"" ("format string")) -> (spreadsheet string=w880:string)
                        n244 = Open/Create/Replace File(file path (use dialog)=w886, error in=w863, operation (0:open)=T6."replace or create with confirmation") -> (refnum out=w881:refnum<file>, error out=w872:errorcluster)  [unwired: 3 in, 1 out]
                        n245 = Write to Text File(file (use dialog)=w881, text=w880, error in=w872) -> (refnum out=w875:refnum<file>, error out=w873:errorcluster)  [unwired: 1 in, 1 out]
                        n246 = Array To Spreadsheet String(delimiter (Tab)=",", array=w874, 3:"%.6f" ("format string")) -> (spreadsheet string=w878:string)
                        n247 = Write to Text File(file (use dialog)=w875, text=w878, error in=w873) -> (refnum out=w877:refnum<file>, error out=w871:errorcluster)  [unwired: 1 in, 1 out]
                        n248 = Close File(refnum=w877, error in=w871) -> (error out=w869:errorcluster)  [unwired: 1 out]
                        n249 = call <vilib>:"Clear Errors.vi"("error in (no error)"=w869, "specific error code to clear (0: all)"=43) -> ("error out"=w868:errorcluster)  [unwired: 4 in, 1 out]
                      }
                    }
                  }
                }
                n250 = invoke class="TrioPC" method="GetAxisVariable"(reference=w173, error in=w209, "Variable"="AXISSTATUS", "Axis"=i16 0) -> (reference out=w208:refnum<k7>, error out=w201:errorcluster, "Value"=w203:dbl)  [unwired: 2 in, 3 out]
                n251 = invoke class="TrioPC" method="GetAxisVariable"(reference=w173, "Variable"="AXISSTATUS", "Axis"=i16 1) -> ("Value"=w202:dbl)  [unwired: 3 in, 5 out]
                n252 = invoke class="TrioPC" method="GetAxisVariable"(reference=w173, "Variable"="AXISSTATUS", "Axis"=i16 2) -> ("Value"=w200:dbl)  [unwired: 3 in, 5 out]
                n253 = call "Controller - Generate Axis Error.vi"("Error Code"=w203) -> ("Error Description"=w193:errorcluster)
                "X Axis Error" <- w193
                n254 = call "Controller - Generate Axis Error.vi"("Error Code"=w202) -> ("Error Description"=w192:errorcluster)
                "Y Axis Error" <- w192
                n255 = call "Controller - Generate Axis Error.vi"("Error Code"=w200) -> ("Error Description"=w197:errorcluster)
                "Z Axis Error" <- w197
                n256 = Unbundle By Name(w193) -> ("status"=→"X Error":bool)
                n257 = Unbundle By Name(w192) -> ("status"=→"Y Error":bool)
                n258 = Unbundle By Name(w197) -> ("status"=→"Z Error":bool)
              }
            }
          }
        }
        "Controller  Error" <- w52
        "Laser Data\nLogging" <- w39
        n259 = To Double Precision Float(number=w53) -> (double precision float=w56:dbl)
        n260 = Divide(x=w56, y=1000.0) -> (x/y=w60:dbl)
        n261 = To Long Integer(number=w60) -> (32bit integer=→"Total Time Elapsed (s)":i32)
        n262 = Array Size(array=w37) -> (size(s)=w38:i32[])
        n263 = Index Array(array=w38) -> (element=→"Laser Data Logged":i32)  [unwired: 1 in]
      }
      n264 = while {
        tunnel: [w1097] -> w15
        tunnel: [w1096] -> w21
        shift-right: [w1088] -> w23
        shift-left: w13 -> [w1092]
        tunnel: errorcluster {"status"=FALSE, "code"=0, "source"=""} ("error in") -> [w1090]
        tunnel: w19 -> [w1091]
        tunnel: [w1087] -> w20
        stop <- w1093 stop-if-true
        n265 = Wait (ms)(milliseconds to wait=u32 200) -> ()  [unwired: 1 out]
        n266 = case shown="True" "Enable Camera" {
          tunnel: [w1099 w1116] -> w1096
          tunnel: [_ w1110] -> w1097
          tunnel: w1092 -> [w1098 w1109]
          tunnel: w1091 -> [_ w1105]
          tunnel: w1090 -> [w1099 w1108]
          tunnel: "Camera Input" -> [w1100 w1104]
          tunnel: [w1098 w1102] -> w1088
          tunnel: [w1100 w1101] -> w1087
          frame False {
          }
          frame True {
            # "Camera"
            n267 = case shown="False" w1109 {
              tunnel: [w1127 w1129] -> w1112
              tunnel: [w1126 w1128] -> w1111
              tunnel: w1108 -> [w1121 w1128]
              tunnel: [w1120 w1130] -> w1106
              tunnel: w1105 -> [w1120 w1130]
              tunnel: w1104 -> [w1119 w1129]
              frame False {
                n268 = call <vilib>:"IMAQdx Open Camera.vi"("error in"=w1121, "Session In"=w1119) -> ("error out"=w1124:errorcluster, "Session Out"=w1125:T3)  [unwired: 1 in, 7 out]
                n269 = call <vilib>:"IMAQdx Read Attributes From String.vi"("error in"=w1124, "Attributes String In"="[NIIMAQ_HEADER]\nType = 2\nVersion = 8\n\n[CAMERA_DATA]\nAcquisitionAttributes::Bayer::Algorithm = \"Bilinear\"\nAcquisitionAttributes::Bayer::GainB = \"1\"\nAcquisitionAttributes::Bayer::GainG = \"1\"\nAcquisitionAttributes::Bayer::GainR = \"1\"\nAcquisitionAttributes::Bayer::Pattern = \"Use hardware value\"\nAcquisitionAttributes::BitsPerPixel = \"Use hardware value\"\nAcquisitionAttributes::HardwareMaximumQueuedBufferCount = \"1000\"\nAcquisitionAttributes::HardwareRequeueBufferListThreshold = \"50\"\nAcquisitionAttributes::IgnoreFirstFrame = \"false\"\nAcquisitionAttributes::ImageDecoderCopyMode = \"Auto\"\nAcquisitionAttributes::OutputImageType = \"Auto\"\nAcquisitionAttributes::OverwriteMode = \"Get Newest\"\nAcquisitionAttributes::PixelSignedness = \"Use hardware value\"\nAcquisitionAttributes::ReceiveTimestampMode = \"None\"\nAcquisitionAttributes::ShiftPixelBits = \"false\"\nAcquisitionAttributes::SwapPixelBytes = \"false\"\nAcquisitionAttributes::Timeout = \"5000\"\nAcquisitionAttributes::VerticalMirror = \"false\"\nAcquisitionAttributes::VideoMode = \"640x480 YUY2 30.00fps\"\nCameraAttributes::BacklightCompensation::Mode = \"Manual\"\nCameraAttributes::BacklightCompensation::Value = \"true\"\nCameraAttributes::Brightness::Mode = \"Manual\"\nCameraAttributes::Brightness::Value = \"0\"\nCameraAttributes::Contrast::Mode = \"Manual\"\nCameraAttributes::Contrast::Value = \"0.179999999999999993\"\nCameraAttributes::Exposure::Mode = \"Auto\"\nCameraAttributes::Gain::Mode = \"Manual\"\nCameraAttributes::Gain::Value = \"1\"\nCameraAttributes::Gamma::Mode = \"Manual\"\nCameraAttributes::Gamma::Value = \"1.5\"\nCameraAttributes::Hue::Mode = \"Manual\"\nCameraAttributes::Hue::Value = \"0\"\nCameraAttributes::Saturation::Mode = \"Manual\"\nCameraAttributes::Saturation::Value = \"8\"\nCameraAttributes::Sharpness::Mode = \"Manual\"\nCameraAttributes::Sharpness::Value = \"3\"\nCameraAttributes::WhiteBalance::Mode = \"Auto\"\n" ("Attributes"), "Session In"=w1125) -> ("error out"=w1122:errorcluster, "Session Out"=w1123:T3)  [unwired: 7 out]
                n270 = call <vilib>:"IMAQdx Configure Grab.vi"("error in"=w1122, "Session In"=w1123) -> ("error out"=w1126:errorcluster, "Session Out"=w1127:T3)  [unwired: 1 in, 7 out]
              }
              frame True {
                # "Camera Initialised"
              }
            }
            n271 = call "IMAQ Create"("Image Name"=w1106) -> ("New Image"=w1107:T1)  [unwired: 3 in, 2 out]
            n272 = call <vilib>:"IMAQdx Grab.vi"("error in"=w1111, "Image In"=w1107, "Session In"=w1112) -> ("error out"=w1113:errorcluster, "Buffer Number Out"=w1114:u32, "Image Out"=w1110:T1, "Session Out"=w1115:T3)  [unwired: 1 in, 4 out]
            "Camera Feed" <- w1110
            n273 = call <vilib>:"Calculate Frames per Second.vi"("Buffer Number"=w1114) -> ()  [unwired: 2 in, 9 out]
            n274 = Unbundle By Name(w1113) -> ("status"=w1103:bool)
            n275 = case shown="True" "Capture Image" {
              tunnel: w1110 -> [_ w1150]
              frame False {
              }
              frame True {
                n276 = local read "Save Directory"() -> (w1146:path)
                n277 = local read "Test Name"() -> (w1148:string)
                n278 = Path To String(path=w1146) -> (string=w1147:string)
                n279 = Concatenate Strings(w1147, "\\" ("string"), w1148, "_photo.jpg" ("string")) -> (w1145:string)
                n280 = String To Path(string=w1145) -> (path=w1142:path)
                n281 = call-poly "IMAQ Write File 2"("File Path"=w1142, "Image"=w1150) -> ("error out"=w1149:errorcluster)  [unwired: 8 in, 1 out]
                n282 = call <vilib>:"Simple Error Handler.vi"("error in (no error)"=w1149) -> ()  [unwired: 4 in, 5 out]
                "Captured Image" <- w1150
              }
            }
            n283 = case "Case Structure_template1" shown="True" w1103 {
              selector: w1103 -> [_ w1136]
              tunnel: [w1133 w1137] -> w1116
              tunnel: w1113 -> [w1133 w1141]
              tunnel: w1115 -> [w1131 w1139]
              tunnel: [TRUE FALSE] -> w1102
              tunnel: [w1131 _] -> w1101
              frame False {
              }
              frame True {
                n284 = Not(x=w1136) -> (.not. x?=w1135:bool)
                n285 = call <vilib>:"IMAQdx Close Camera.vi"("error in"=w1141, "Session In"=w1139) -> ("error out"=w1140:errorcluster)  [unwired: 9 out]
                n286 = local write "Enable Camera"(w1135) -> ()
                n287 = call <vilib>:"Simple Error Handler.vi"("error in (no error)"=w1140) -> ("error out"=w1138:errorcluster)  [unwired: 4 in, 4 out]
                n288 = call <vilib>:"Clear Errors.vi"("error in (no error)"=w1138) -> ("error out"=w1137:errorcluster)  [unwired: 5 in, 1 out]
              }
            }
          }
        }
        n289 = local read "STOP"() -> (w1093:bool)
      }
      n290 = while {
        shift-right: [w899] -> _
        shift-left: w29 -> [w913]
        shift-right: [w911] -> _
        shift-left: w28 -> [w912]
        shift-right: [w907] -> _
        shift-left: w27 -> [w909]
        shift-right: [w905] -> _
        shift-left: w26 -> [w906]
        shift-right: [w894] -> _
        shift-left: errorcluster {"status"=FALSE, "code"=0, "source"=""} ("error constant") -> [w904]
        shift-right: [w903] -> _
        shift-left: w24 -> [w902]
        stop <- w898 stop-if-true
        w910 = 0.05  # target time
        n291 = call "Elapsed Time"("Time Target (s)"=w910, "Reset"=w909) -> ("Time has Elapsed"=w908:bool)  [unwired: 10 in, 7 out]
        n292 = case shown="\"Save\"" w913 {
          tunnel: w912 -> [w921 w931 _ w967 w986 w1034 w1059 _]
          tunnel: w904 -> [w915 w927 w956 w970 w989 w1020 w1062 w1080]
          tunnel: [w921 w931 w952 w967 w986 w1034 w1059 T9 {"addInfo"={"triggerCount"=0, "pulseCount"=0}, "outMeasurementData"=[]} ("KEYENCE_MEASUREMENT_DATA")] -> w911
          tunnel: [w918 w929 w955 Sensor_Station_States."Log" ("Next State") w982 w1025 w1060 w1074] -> w901
          tunnel: w908 -> [_ _ _ _ _ _ w1061 _]
          tunnel: [_ _ w958 _ _ _ _ _] -> w907
          tunnel: w906 -> [w914 w928 w957 w969 w990 w1023 w1064 _]
          tunnel: [w914 w928 w957 w969 w988 w1023 w1064 FALSE ("Chromatic Logging?")] -> w905
          tunnel: [w915 w923 w953 w970 w979 w1021 w1062 errorcluster {"status"=FALSE, "code"=0, "source"=""} ("error constant")] -> w894
          tunnel: [w922 w924 w951 w971 w987 w1024 w1063 FALSE] -> w903
          tunnel: w902 -> [w922 _ w951 w971 w987 w1024 w1063 w1073]
          tunnel: [_ _ _ _ _ _ _ w1071] -> w898
          tunnel: "Enable Chromatic" -> [w917 w925 _ _ _ _ w1058 _]
          tunnel: "Chromatic Data \nLogging" -> [_ _ _ _ w981 _ _ _]
          frame "Idle", Default {
            w920 = Sensor_Station_States."Initialise"  # Next State
            n293 = Wait (ms)(milliseconds to wait=u32 200) -> ()  [unwired: 1 out]
            n294 = Select(t=w920, s=w917, f=Sensor_Station_States."Idle" ("Next State")) -> (s? t:f=w918:T7)
          }
          frame "Initialise" {
            w930 = Sensor_Station_States."Acquire"  # Next State
            # "Initialise Chromatic Confocal"
            n295 = case shown="True" w925 {
              tunnel: [w932 w937] -> w923
              tunnel: [FALSE w936] -> w924
              tunnel: w927 -> [w932 w938]
              frame False {
              }
              frame True {
                n296 = local read "IP Address"() -> (w940:u8[])
                n297 = call <vilib>:"Clear Errors.vi"("error in (no error)"=w938) -> ("error out"=w934:errorcluster)  [unwired: 5 in, 1 out]
                n298 = Index Array(array=w940) -> (element #1=w945:u8, element #2=w946:u8, element #3=w947:u8, element #4=w948:u8)  [unwired: 4 in]
                n299 = local read "Port"() -> (w939:u32)
                n300 = Bundle("IP Address"=w945, "IP Address"=w946, "IP Address"=w947, "IP Address"=w948) -> (w949:T14)  [unwired: 1 in]
                n301 = local read "Timeout"() -> (w941:u32)
                n302 = local read "Comm Interface"() -> (w942:enum8{"USB", "ETHERNET"})
                n303 = local read "Device ID"() -> (w943:i32)
                n304 = Bundle By Name(cluster=T8 {"IP Address"={"IP1"=0, "IP2"=0, "IP3"=0, "IP4"=0}, "portNo"=0} ("ethernetSetting"), "IP Address"=w949, "portNo"=w939) -> (w950:T8)
                n305 = call "Initialize.vi"("Comm Interface"=w942, "error in (no error)"=w934, "ethernetSetting"=w950, "timeout"=w941, "deviceId"=w943) -> ("error out"=w937:errorcluster)  [unwired: 6 in]
                n306 = Unbundle By Name(w937) -> ("status"=w935:bool)
                n307 = Not(x=w935) -> (.not. x?=w936:bool)
              }
            }
            n308 = local write "Enable Chromatic"(w924) -> ()
            n309 = Select(t=w930, s=w924, f=Sensor_Station_States."Idle" ("Next State")) -> (s? t:f=w929:T7)
          }
          frame "Acquire" {
            w955 = Sensor_Station_States."Visualise"  # Next State
            w958 = TRUE  # Reset Elapsed Time counter
            n310 = local read "Device ID"() -> (w954:i32)
            n311 = call "CL3IF_GetMeasurementData.vi"("error in"=w956, "deviceId"=w954) -> ("error out"=w953:errorcluster, "MEASUREMENT_DATA"=w952:T9)  [unwired: 8 in]
          }
          frame "Visualise" {
            n312 = Unbundle By Name(w967) -> ("outMeasurementData"=w965:T10[])
            n313 = Index Array(array=w965, index=0) -> (element=w964:T10)
            n314 = for {
              tunnel: w965 -> [w978] mode=indexing
              tunnel: [w977] -> w966 mode=indexing
              i -> [w976]
              n315 = Unbundle By Name(w978) -> ("measurementValue"=w972:i32, "valueInfo"=w974:T11, "judgeResult"=w973:T12)
              n316 = Increment(x=w976) -> (x+1=w975:i32)
              n317 = Bundle(w975, "measurementValue"=w972, "valueInfo"=w974, "judgeResult"=w973) -> (w977:T15)  [unwired: 1 in]
            }
            "Measurement Data" <- w966
            n318 = Unbundle By Name(w964) -> ("measurementValue"=w963:i32)
            n319 = To Double Precision Float(number=w963) -> (double precision float=w959:dbl)
            n320 = Divide(x=w959, y=1000.0) -> (x/y=→"Chromatic Confocal":dbl)
          }
          frame "Log" {
            w984 = Sensor_Station_States."Save"  # Next State
            n321 = local read "Device ID"() -> (w980:i32)
            n322 = case shown="False" w981 {
              tunnel: w990 -> [w995 w1009]
              tunnel: w989 -> [w996 w1008]
              tunnel: [w994 w1007] -> w979
              tunnel: [FALSE TRUE] -> w988
              tunnel: [w992 FALSE ("conSaveData")] -> w985
              tunnel: w980 -> [w991 w1004]
              frame False {
                n323 = case shown="True" w995 {
                  tunnel: w996 -> [w998 w1002]
                  tunnel: [w998 w1000] -> w994
                  tunnel: [FALSE ("conSaveData") TRUE ("conSaveData")] -> w992
                  tunnel: w991 -> [_ w999]
                  frame False {
                    # "Not Logging\nDo nothing"
                  }
                  frame True {
                    # "Move to Save State"
                    # "Stop Logging & Record Data Index"
                    n324 = call "CL3IF_GetTrendIndex.vi"("error in"=w1002, "deviceId"=w999) -> ("error out"=w1000:errorcluster, "index"=→"Index End":u32)  [unwired: 8 in]
                  }
                }
              }
              frame True {
                n325 = case shown="False" w1009 {
                  tunnel: w1008 -> [w1012 w1014]
                  tunnel: [w1011 w1014] -> w1007
                  tunnel: w1004 -> [w1010 _]
                  frame False {
                    # "Start Logging"
                    n326 = call "CL3IF_GetTrendIndex.vi"("error in"=w1012, "deviceId"=w1010) -> ("error out"=w1011:errorcluster, "index"=→"Index Start":u32)  [unwired: 8 in]
                  }
                  frame True {
                    # "Currently Logging\nDo nothing"
                  }
                }
              }
            }
            n327 = Select(t=w984, s=w985, f=Sensor_Station_States."Check Time" ("Next State")) -> (s? t:f=w982:T7)
          }
          frame "Save" {
            w1025 = Sensor_Station_States."Check Time"  # Next State
            n328 = local read "Save Directory"() -> (w1031:path)
            n329 = local read "Index Start"() -> (w1033:u32)
            n330 = local read "Index End"() -> (w1032:u32)
            n331 = local read "Test Name"() -> (w1028:string)
            n332 = local read "Suffix"() -> (w1015:string)
            n333 = local read "Device ID"() -> (w1022:i32)
            n334 = Path To String(path=w1031) -> (string=w1030:string)
            n335 = Concatenate Strings(w1030, "\\" ("string"), w1028, w1015, "_confocal.csv" ("string")) -> (w1027:string)
            n336 = Subtract(x=w1032, y=w1033) -> (x-y=w1041:u32)
            "Chromatic Data Logged" <- w1041
            n337 = String To Path(string=w1027) -> (path=w1026:path)
            n338 = call "CL3IF_GetTrendData.vi"("requestDataCount"=w1041, "index"=w1033, "deviceId"=w1022) -> ("measurementData"=w1040:T9[])  [unwired: 4 in, 4 out]
            n339 = Open/Create/Replace File(file path (use dialog)=w1026, operation (0:open)=T6."replace or create with confirmation") -> (refnum out=w1039:refnum<file>, error out=w1036:errorcluster)  [unwired: 4 in, 1 out]
            n340 = for {
              tunnel: w1040 -> [w1057] mode=indexing
              tunnel: w1039 -> [w1046]
              tunnel: [w1044] -> w1038
              tunnel: w1036 -> [w1043]
              tunnel: [w1042] -> w1035
              n341 = Unbundle By Name(w1057) -> ("outMeasurementData"=w1055:T10[])
              n342 = Index Array(array=w1055, index=0) -> (element=w1054:T10)
              n343 = Unbundle By Name(w1054) -> ("measurementValue"=w1051:i32)
              n344 = To Double Precision Float(number=w1051) -> (double precision float=w1052:dbl)
              n345 = Divide(x=w1052, y=1000.0) -> (x/y=w1050:dbl)
              n346 = Format Into String(format string="%.6f%s", error in=w1043, w1050, "\r\n") -> (resulting string=w1047:string, error out=w1045:errorcluster)  [unwired: 1 in]
              n347 = Write to Text File(file (use dialog)=w1046, text=w1047, error in=w1045) -> (refnum out=w1044:refnum<file>, error out=w1042:errorcluster)  [unwired: 1 in, 1 out]
            }
            n348 = Close File(refnum=w1038, error in=w1035) -> (error out=w1018:errorcluster)  [unwired: 1 out]
            n349 = call <vilib>:"Clear Errors.vi"("error in (no error)"=w1018, "specific error code to clear (0: all)"=43) -> ("error out"=w1017:errorcluster)  [unwired: 4 in, 1 out]
            n350 = Merge Errors(w1017, w1020) -> (w1021:errorcluster)
          }
          frame "Check Time" {
            n351 = case shown="True" w1058 {
              tunnel: w1061 -> [_ w1068]
              tunnel: [w1066 w1067] -> w1060
              frame False {
                w1066 = Sensor_Station_States."Close"  # Next State
                # "Close Chromatic Connection"
              }
              frame True {
                w1069 = Sensor_Station_States."Acquire"  # Next State
                # "Wait Until Target Time Elapsed"
                n352 = Select(t=w1069, s=w1068, f=Sensor_Station_States."Check Time" ("Next State")) -> (s? t:f=w1067:T7)
              }
            }
            n353 = Wait (ms)(milliseconds to wait=u32 10) -> ()  [unwired: 1 out]
          }
          frame "Close" {
            w1076 = Sensor_Station_States."Close"  # Not Used
            n354 = case shown="True" w1073 {
              tunnel: w1080 -> [_ w1082]
              frame False {
              }
              frame True {
                n355 = local read "Device ID"() -> (w1081:i32)
                n356 = call "Close.vi"("error in (no error)"=w1082, "deviceId"=w1081) -> ()  [unwired: 9 in, 1 out]
              }
            }
            n357 = local read "STOP"() -> (w1071:bool)
            n358 = Select(t=w1076, s=w1071, f=Sensor_Station_States."Idle" ("Next State")) -> (s? t:f=w1074:T7)
          }
        }
        "Chromatic Sensor Error" <- w894
        n359 = local read "STOP"() -> (w895:bool)
        n360 = Select(t=Sensor_Station_States."Close" ("Next State"), s=w895, f=w901) -> (s? t:f=w899:T7)
      }
      n361 = call "Imaq Dispose"("Image"=w15) -> ()  [unwired: 5 in, 1 out]
      n362 = case shown="True" w23 {
        tunnel: w20 -> [_ w1086]
        tunnel: w21 -> [w1083 w1084]
        tunnel: [w1083 w1085] -> w22
        frame False {
        }
        frame True {
          n363 = call <vilib>:"IMAQdx Close Camera.vi"("error in"=w1084, "Session In"=w1086) -> ("error out"=w1085:errorcluster)  [unwired: 9 out]
        }
      }
      n364 = call <vilib>:"Simple Error Handler.vi"("error in (no error)"=w22) -> ()  [unwired: 4 in, 5 out]
    }
    frame #2 {
      n365 = call-poly <vilib>:"Close Input Device.vi"("device ID"=w1161) -> ()  [unwired: 9 in, 1 out]
      n366 = invoke class="TrioPC" method="Execute"(reference=w1159, error in=w1160, "Command"="RAPIDSTOP(2)") -> (reference out=w1155:refnum<k7>, error out=w1156:errorcluster)  [unwired: 1 in, 2 out]
      n367 = invoke class="TrioPC" method="SetVariable"(reference=w1155, error in=w1156, "Variable"="WDOG", "Value"=0.0) -> (reference out=w1154:refnum<k7>, error out=w1153:errorcluster)  [unwired: 1 in, 3 out]
      n368 = invoke class="TrioPC" method="Close"(reference=w1154, error in=w1153) -> (reference out=w1162:refnum<k7>, error out=w1163:errorcluster)  [unwired: 2 in, 2 out]
      n369 = Close Reference(reference=w1162, error in (no error)=w1163) -> (error out=w1158:errorcluster)
      n370 = call <vilib>:"Simple Error Handler.vi"("error in (no error)"=w1158) -> ()  [unwired: 4 in, 5 out]
    }
  }
